vi "eventMode.vi"() -> ()   [LabVIEW 2019]
uses:
  TypeDefs/pixArrSmol.ctl
  <vilib>/Math Plots/3D Math Plots/3D Surface/3D Surface XCtrl/3D Surface.xctl
  <vilib>/Instr/_visa.llb/VISA Flush IO Buffer Mask.ctl
  <extravilib>/ChannelInstances/Tag-bool/Read With Abort.vi
  <extravilib>/ChannelInstances/Tag-bool/Write With Abort.vi
  <extravilib>/ChannelInstances/Tag-bool/Instantiate.vi
  <extravilib>/ChannelInstances/Tag-bool/EndpointRead.vi
  <extravilib>/ChannelInstances/Tag-bool/Endpoint.vi
  <vilib>/Instr/_visa.llb/VISA Configure Serial Port (Instr).vi
  <extravilib>/ChannelInstances/Tag-bool.lvlib
  TypeDefs/serialSettings_Global.vi
panel:
  in  "Reset EEPROM":bool
  in  "Update EEPROM":bool
  in  "Serial Settings":T1={"VISA resource name"="COM6", "baud rate"=115200, "data bits"=8, "parity"=enum."None", "stop bits"=10, "flow control"=0} {"baud rate" items=["75"=75, "110"=110, "134"=134, "150"=150, "300"=300, "600"=600, "1200"=1200, "1800"=1800, "2400"=2400, "4800"=4800, "7200"=7200, "9600"=9600, "14400"=14400, "19200"=19200, "28800"=28800, "38400"=38400, "56000"=56000, "57600"=57600, "115200"=115200, "128000"=128000, "230400"=230400]; "stop bits" items=["1.0"=10, "1.5"=15, "2.0"=20]; "flow control" items=["None"=0, "XON/XOFF"=1, "RTS/CTS"=2, "DTR/DSR"=4]}
  out "Serial2 Same?":bool caption="Match 2?"
  out "Serial1 Same?":bool caption="Match?"
  in  "CZT 2 Serial In":u32 caption="Enter CZT 2 Serial Number"
  out "CZT 2 Serial":sgl=nan
  in  "CZT 1 Serial In":u32 caption="Enter CZT 1 Serial Number"
  out "CZT 1 Serial":sgl=nan
  in  "Clear Serial":bool
  in  "Read Serial":bool
  in  "Iteration Limit":u32=4999
  out "Exit error code":errorcluster
  in  "Event Counts":enum32{"3D Surface ", "Histogram", "Heat Map"}(tab)
  out "Detector Surface":refnum<class "3D Plot Datatype.lvclass">[](xcontrol)
  out "Event Count Histogram":T2(graph)
  out "Intensity Graph":u32[][](graph)
  out "Energy Spectrum":T2(graph)
  out "Input Size":i32[](array[numeric])
  out "All rows":string[][](array[string])
  out "Clean No Dups Size":i32[](array[numeric])
  out "Clean+No Dups":string[][](array[string])
  in  "Select CZT":enum32{"CZT 1", "CZT 2"}(radio)
  in  "PixOff":bool
  in  "Get All Pixel Status":bool
  out "Column":u8=1
  out "Row":string="A"
  in  "PixOn":bool
  in  "Choose Pixel":u8 format="%02.0f"
  in  "CZT Tabs":enum32{"CZT 1", "CZT 2"}(tab)=enum."CZT 2"
  out "Pixel Status 1":T3=[[TRUE, TRUE, TRUE, TRUE, TRUE, TRUE, TRUE, TRUE, TRUE, TRUE, TRUE, TRUE, TRUE, TRUE, TRUE, TRUE, TRUE], [TRUE, TRUE, TRUE, TRUE, TRUE, TRUE, TRUE, TRUE, TRUE, TRUE, TRUE, TRUE, TRUE, TRUE, TRUE, TRUE, TRUE], [TRUE, TRUE, TRUE, TRUE, TRUE, TRUE, TRUE, TRUE, TRUE, TRUE, TRUE, TRUE, TRUE, TRUE, TRUE, TRUE, TRUE], [TRUE, TRUE, TRUE, TRUE, TRUE, TRUE, TRUE, TRUE, TRUE, TRUE, TRUE, TRUE, TRUE, TRUE, TRUE, TRUE, TRUE], [TRUE, TRUE, TRUE, TRUE, TRUE, TRUE, TRUE, TRUE, TRUE, TRUE, TRUE, TRUE, TRUE, TRUE, TRUE, TRUE, TRUE], [TRUE, TRUE, TRUE, TRUE, TRUE, TRUE, TRUE, TRUE, TRUE, TRUE, TRUE, TRUE, TRUE, TRUE, TRUE, TRUE, TRUE], [TRUE, TRUE, TRUE, TRUE, TRUE, TRUE, TRUE, TRUE, TRUE, TRUE, TRUE, TRUE, TRUE, TRUE, TRUE, TRUE, TRUE], [TRUE, TRUE, TRUE, TRUE, TRUE, TRUE, TRUE, TRUE, TRUE, TRUE, TRUE, TRUE, TRUE, TRUE, TRUE, TRUE, TRUE], [TRUE, TRUE, TRUE, TRUE, TRUE, TRUE, TRUE, TRUE, TRUE, TRUE, TRUE, TRUE, TRUE, TRUE, TRUE, TRUE, TRUE], [TRUE, TRUE, TRUE, TRUE, TRUE, TRUE, TRUE, TRUE, TRUE, TRUE, TRUE, TRUE, TRUE, TRUE, TRUE, TRUE, TRUE], [TRUE, TRUE, TRUE, TRUE, TRUE, TRUE, TRUE, TRUE, TRUE, TRUE, TRUE, TRUE, TRUE, TRUE, TRUE, TRUE, TRUE], [TRUE, TRUE, TRUE, TRUE, TRUE, TRUE, TRUE, TRUE, TRUE, TRUE, TRUE, TRUE, TRUE, TRUE, TRUE, TRUE, TRUE], [TRUE, TRUE, TRUE, TRUE, TRUE, TRUE, TRUE, TRUE, TRUE, TRUE, TRUE, TRUE, TRUE, TRUE, TRUE, TRUE, TRUE], [TRUE, TRUE, TRUE, TRUE, TRUE, TRUE, TRUE, TRUE, TRUE, TRUE, TRUE, TRUE, TRUE, TRUE, TRUE, TRUE, TRUE], [TRUE, TRUE, TRUE, TRUE, TRUE, TRUE, TRUE, TRUE, TRUE, TRUE, TRUE, TRUE, TRUE, TRUE, TRUE, TRUE, TRUE], [TRUE, TRUE, TRUE, TRUE, TRUE, TRUE, TRUE, TRUE, TRUE, TRUE, TRUE, TRUE, TRUE, TRUE, TRUE, TRUE, TRUE]]
  out "Pixel Status 2":T3=[[TRUE, TRUE, TRUE, TRUE, TRUE, TRUE, TRUE, TRUE, TRUE, TRUE, TRUE, TRUE, TRUE, TRUE, TRUE, TRUE, TRUE], [TRUE, TRUE, TRUE, TRUE, TRUE, TRUE, TRUE, TRUE, TRUE, TRUE, TRUE, TRUE, TRUE, TRUE, TRUE, TRUE, TRUE], [TRUE, TRUE, TRUE, TRUE, TRUE, TRUE, TRUE, TRUE, TRUE, TRUE, TRUE, TRUE, TRUE, TRUE, TRUE, TRUE, TRUE], [TRUE, TRUE, TRUE, TRUE, TRUE, TRUE, TRUE, TRUE, TRUE, TRUE, TRUE, TRUE, TRUE, TRUE, TRUE, TRUE, TRUE], [TRUE, TRUE, TRUE, TRUE, TRUE, TRUE, TRUE, TRUE, TRUE, TRUE, TRUE, TRUE, TRUE, TRUE, TRUE, TRUE, TRUE], [TRUE, TRUE, TRUE, TRUE, TRUE, TRUE, TRUE, TRUE, TRUE, TRUE, TRUE, TRUE, TRUE, TRUE, TRUE, TRUE, TRUE], [TRUE, TRUE, TRUE, TRUE, TRUE, TRUE, TRUE, TRUE, TRUE, TRUE, TRUE, TRUE, TRUE, TRUE, TRUE, TRUE, TRUE], [TRUE, TRUE, TRUE, TRUE, TRUE, TRUE, TRUE, TRUE, TRUE, TRUE, TRUE, TRUE, TRUE, TRUE, TRUE, TRUE, TRUE], [TRUE, TRUE, TRUE, TRUE, TRUE, TRUE, TRUE, TRUE, TRUE, TRUE, TRUE, TRUE, TRUE, TRUE, TRUE, TRUE, TRUE], [TRUE, TRUE, TRUE, TRUE, TRUE, TRUE, TRUE, TRUE, TRUE, TRUE, TRUE, TRUE, TRUE, TRUE, TRUE, TRUE, TRUE], [TRUE, TRUE, TRUE, TRUE, TRUE, TRUE, TRUE, TRUE, TRUE, TRUE, TRUE, TRUE, TRUE, TRUE, TRUE, TRUE, TRUE], [TRUE, TRUE, TRUE, TRUE, TRUE, TRUE, TRUE, TRUE, TRUE, TRUE, TRUE, TRUE, TRUE, TRUE, TRUE, TRUE, TRUE], [TRUE, TRUE, TRUE, TRUE, TRUE, TRUE, TRUE, TRUE, TRUE, TRUE, TRUE, TRUE, TRUE, TRUE, TRUE, TRUE, TRUE], [TRUE, TRUE, TRUE, TRUE, TRUE, TRUE, TRUE, TRUE, TRUE, TRUE, TRUE, TRUE, TRUE, TRUE, TRUE, TRUE, TRUE], [TRUE, TRUE, TRUE, TRUE, TRUE, TRUE, TRUE, TRUE, TRUE, TRUE, TRUE, TRUE, TRUE, TRUE, TRUE, TRUE, TRUE], [TRUE, TRUE, TRUE, TRUE, TRUE, TRUE, TRUE, TRUE, TRUE, TRUE, TRUE, TRUE, TRUE, TRUE, TRUE, TRUE, TRUE]]
  out "Noisy Pixel List":i32[][](array[numeric])
  in  "Open CSV":bool
  out "States Left":string
  out "Current Time":timestamp format="%<%x\n%X>T"
  out "CZT 2 \nFrequency":u8 format="%d Mhz"
  in  "Set Clock":bool
  in  "Set CZT Clock":u8(ring)=2 items=["30 Mhz"=6, "25 Mhz"=5, "20 Mhz"=4, "15 Mhz"=3, "10 Mhz"=2]
  out "CZT 1\nFrequency":u8 format="%d Mhz"
  out "CZT 2 Thresh":u16 format="%u KeV"
  in  "Select Threshold Value":u16(slide)=20 min=20 max=200 scale=20.0..200.0
  in  "Set Threshold":bool
  out "CZT 1 Thresh":u16 format="%u KeV"
  in  "Test Description":string caption="(Inserted in FITS header)"
  in  "Stop":bool
  in  "Start Event":bool
  in  "Short Description":string caption="(Appended to file name)"
  in  "User Name":string
  in  "Acquisition Period":T4={"Hours"=0, "Minutes"=0, "Seconds"=10}
  out "Event Mode":bool
  out "Events Count":u32
  out "FITS File":bool
  out "Time elapsed":dbl format="%<%H:%M:%S>t"
  in  "Exit":bool
  # "Event Mode Test"
  # "Event Start:    A0FF55\nEvent Stop:    A00055\nEmu +Eve :    A1FF55\nRead Serial:   BXXX55\nClock Set  :    C00X55\nThresh Set:    EXXX55\nUpdate EE:     F00155\nReset EE   :     F00055"
  # "Pix On  CZT1: D0XX55\nPix Off  CZT1: D1XX55\nPix On  CZT2: D2XX55\nPix Off  CZT2: D3XX55\nChck All Pix  : DFXX55"
  # "Pixel Matrix Settings"
  # "Channel"
  # "Counts"
  # "Energy Threshold Settings"
  # "KeV"
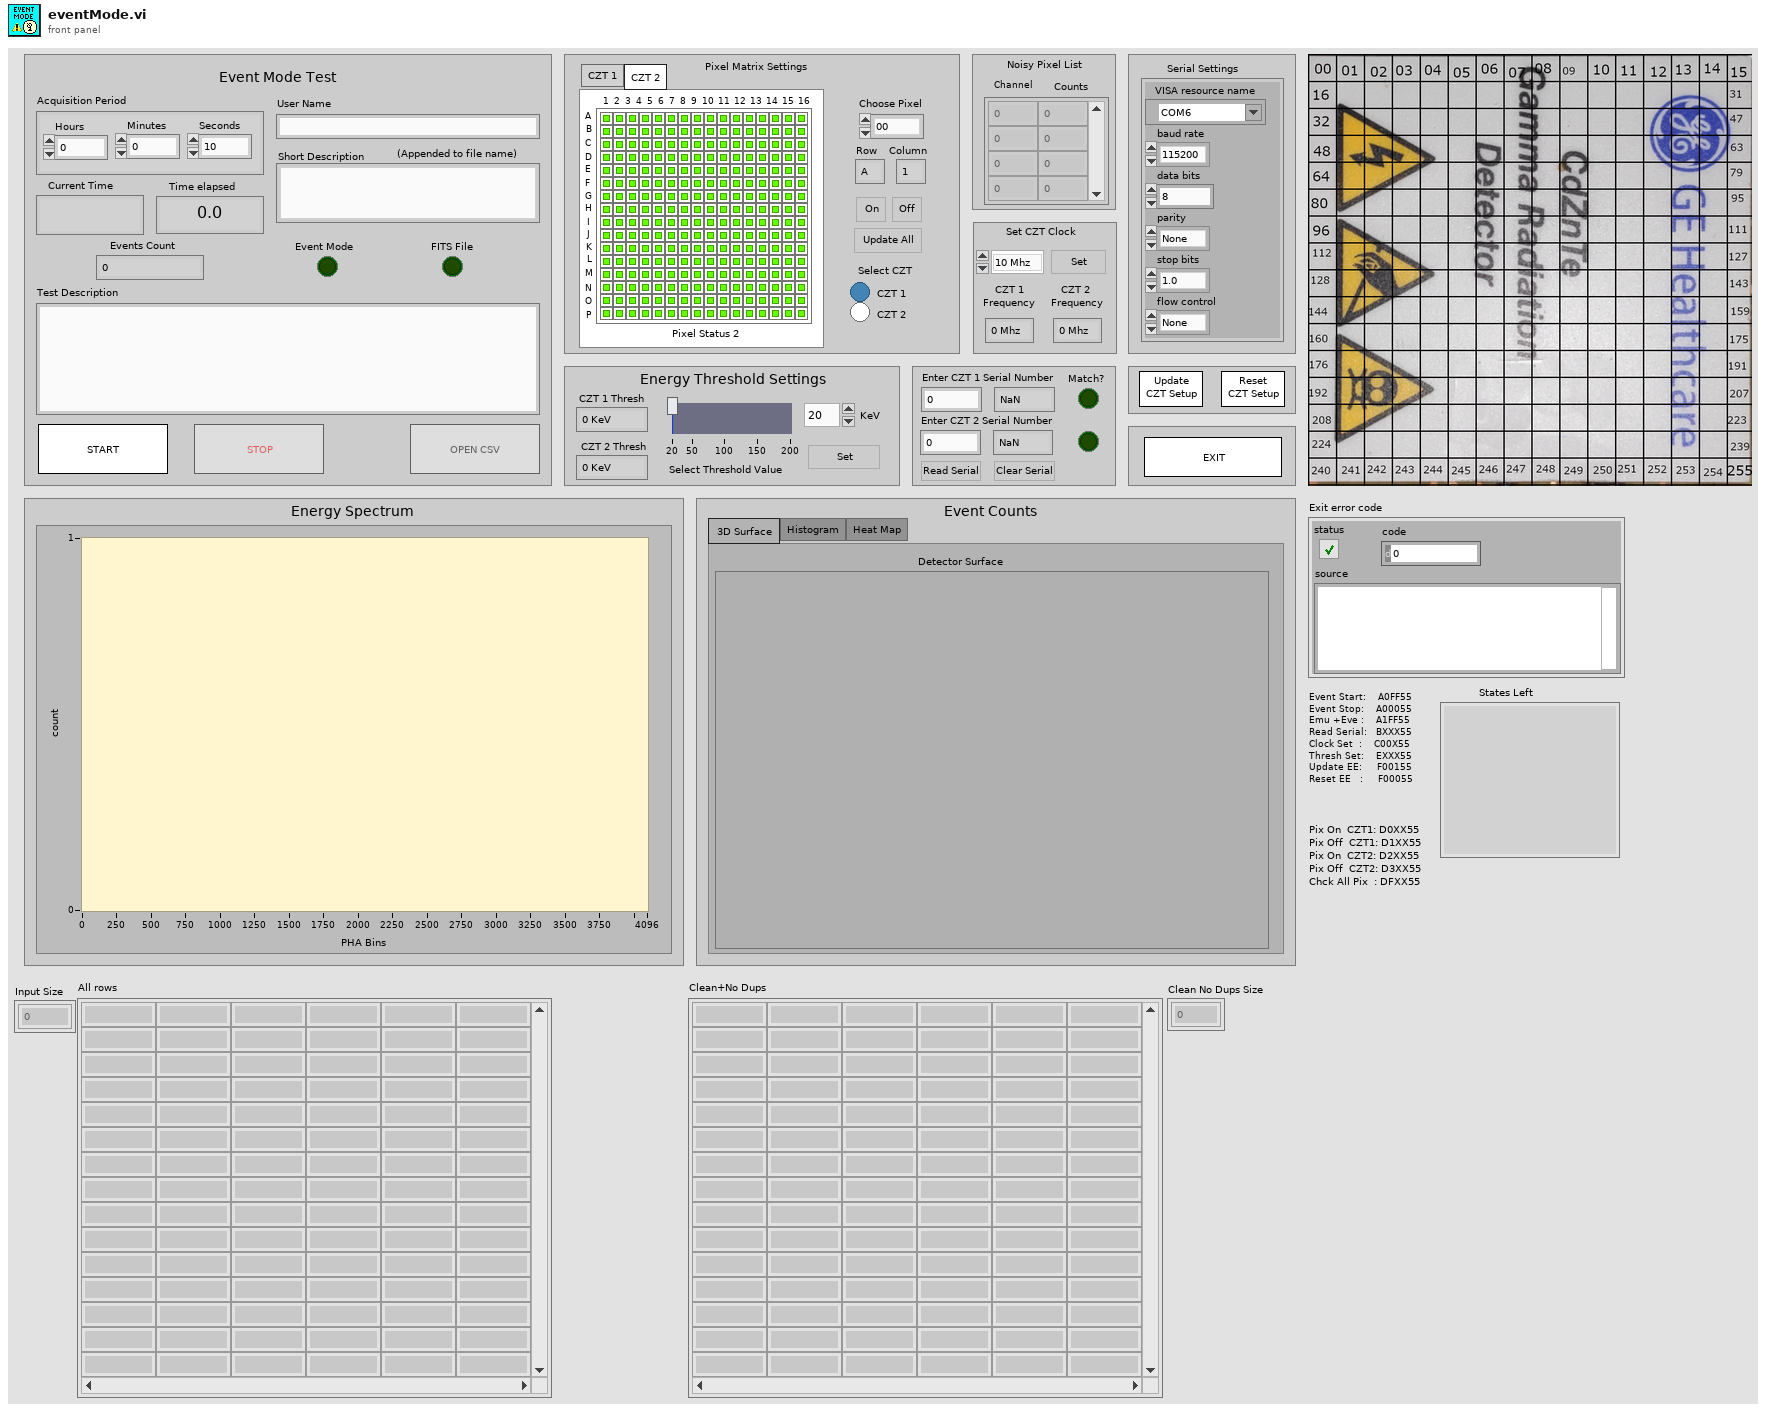
[diagram p1: front panel]
types:
  T1 = cluster{"VISA resource name":refnum<visa-resource-name>, "baud rate":u32, "data bits":u16, "parity":enum16{"None", "Odd", "Even", "Mark", "Space"}, "stop bits":u16, "flow control":u16}
  T2 = cluster{"X Values":dbl[], "Histogram: h(x)":i32[]}
  T3 = typedef "pixArrSmol.ctl" = bool[][]
  T4 = cluster{"Hours":u32, "Minutes":u32, "Seconds":u32}
  T5 = enum32{"Invalid", "Standard", "Closed", "Hidden", "Minimized", "Maximized"}
  T6 = enum32{"invalid app kind", "Development System", "Run Time System", "Student Edition", "Embedded LabVIEW", "Evaluation", "Custom"}
  T7 = enum8{"Enabled", "Disabled", "Disabled and Grayed Out"}
  T8 = typedef "Tag-bool.lvlib/))Channel.ctl" = refnum<queue>
  T9 = cluster{"Core":cluster{"Current VI Reference":refnum<vi>, "Close Panel on Exit?":bool}, "Stop Pressed?":bool, "Start Time":dbl, "Acquisition Period":dbl, "Iteration Count":u32, "CSV File Data":cluster{"Dump txt file path":path, "Data Buffer":string, "Valid Data in Buffer":i32, "CSV file path":path, "Fits File name":string, "Test Start time":timestamp}, "User & Config Data":cluster{"User Name":string, "Short Description":string, "Description":string, "CZT Threshold 1":u16, "CZT Threshold 2":u16}, "Pixel Status 1":cluster{"Pixel Number":u16, "Pixel En/Dis?":bool, "Pixel Array":bool[][], "Disabled Pixels":u8[]}, "Pixel Status 2":cluster{"Pixel Number":u16, "Pixel En/Dis?":bool, "Pixel Array":bool[][], "Disabled Pixels":u8[]}}
  T10 = cluster{"Pixel Number":u16, "Pixel En/Dis?":bool, "Pixel Array":bool[][], "Disabled Pixels":u8[]}
  T11 = cluster{"User Name":string, "Short Description":string, "Description":string, "CZT Threshold 1":u16, "CZT Threshold 2":u16}
  T12 = cluster{"Dump txt file path":path, "Data Buffer":string, "Valid Data in Buffer":i32, "CSV file path":path, "Fits File name":string, "Test Start time":timestamp}
  T13 = cluster{"Current VI Reference":refnum<vi>, "Close Panel on Exit?":bool}
  T14 = cluster{"User Name":string, "Short Description ":string, "Test Description":string, "Value":u16, "Value":u16}
  T15 = cluster{"Dump txt file path":path, "Data buffer OUT":string, "Valid Data Buf OUT":i32, "CSV file path":path, "Fits File name":string, "Test Start time":timestamp}
  T16 = typedef "VISA Flush IO Buffer Mask.ctl" = u16
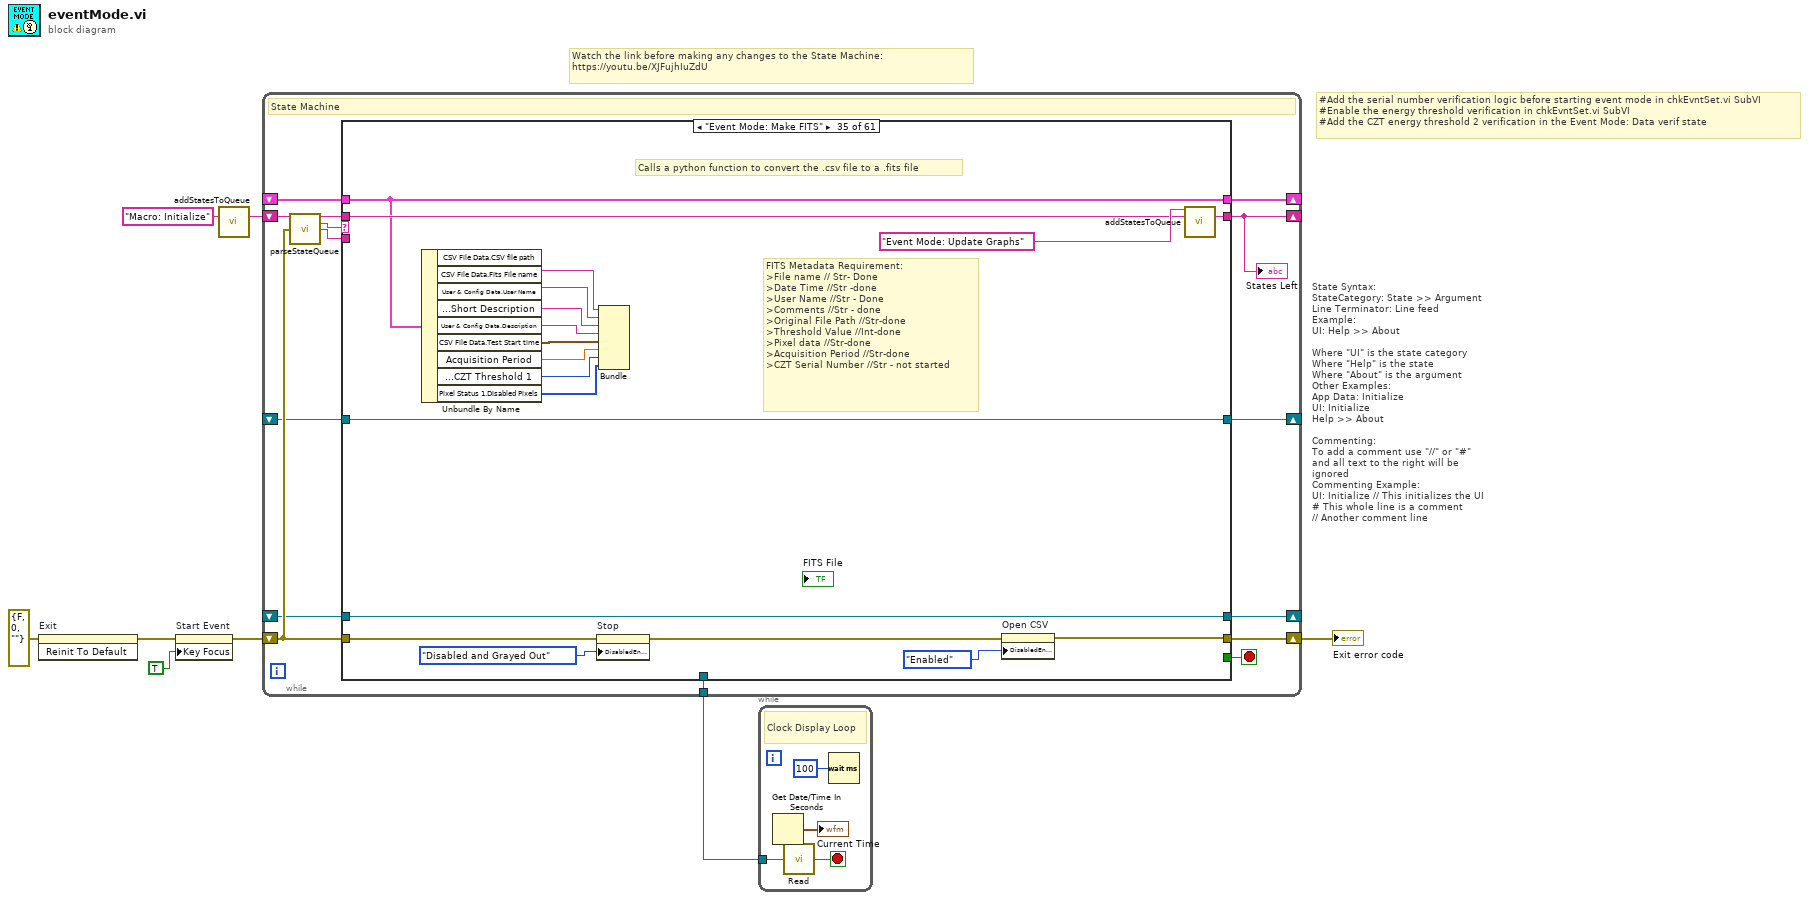
[diagram p0: block diagram]
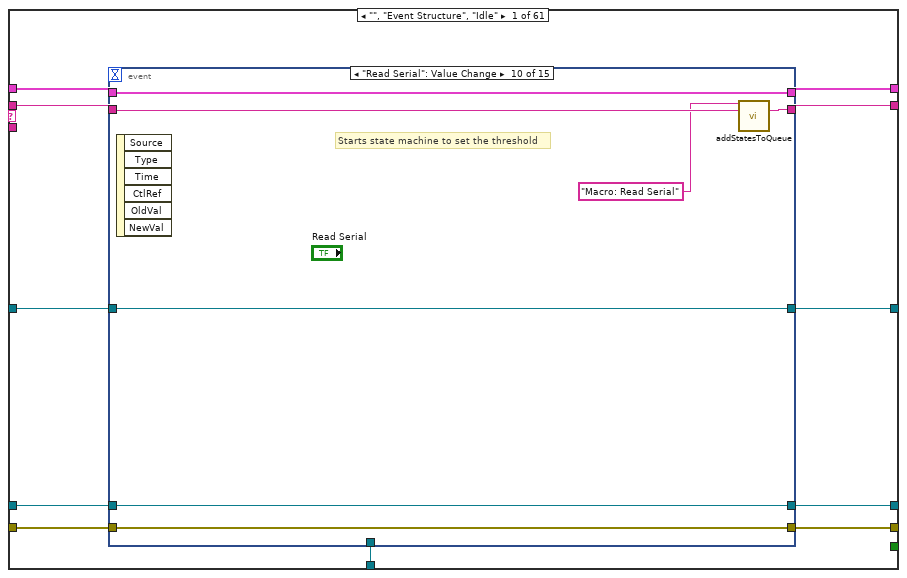
[diagram p2: hidden frame]
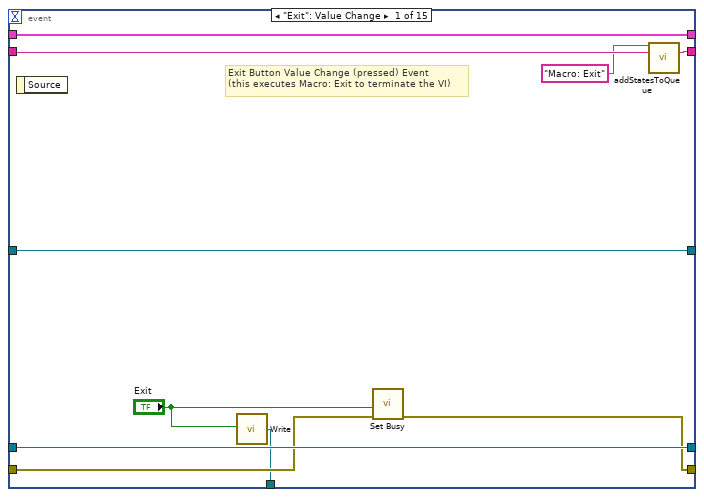
[diagram p3: hidden frame]
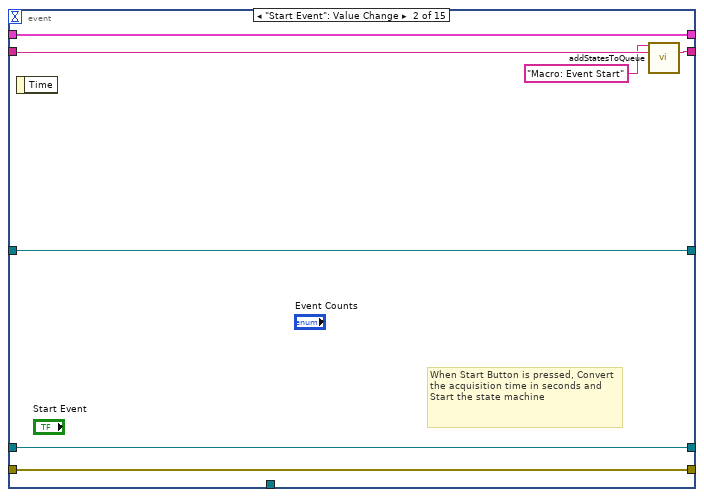
[diagram p4: hidden frame]
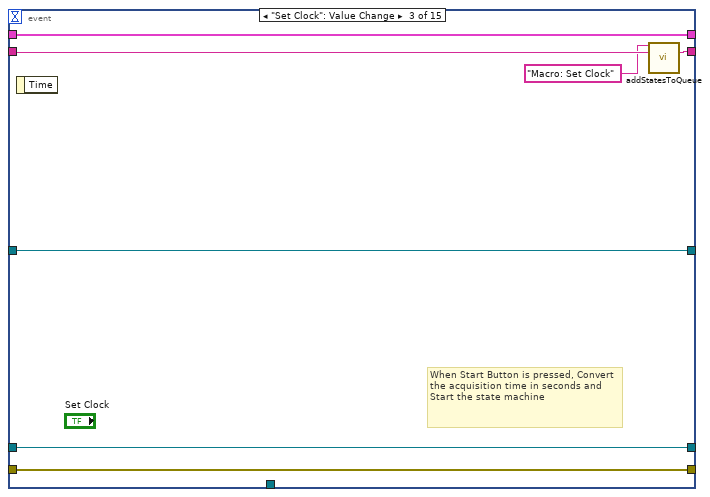
[diagram p5: hidden frame]
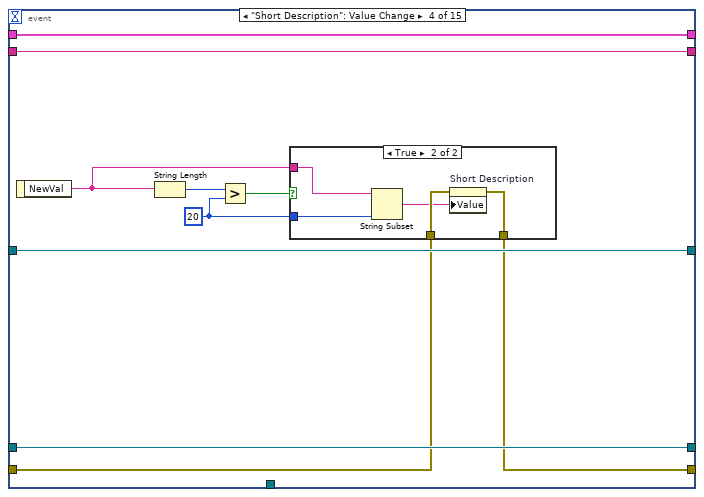
[diagram p6: hidden frame]
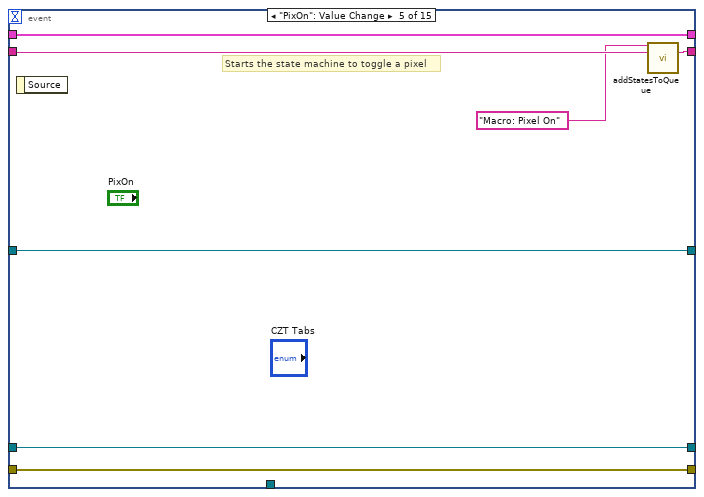
[diagram p8: hidden frame]
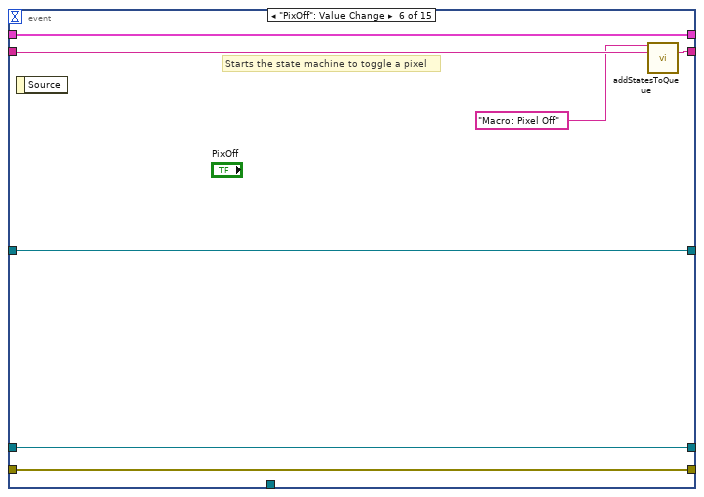
[diagram p9: hidden frame]
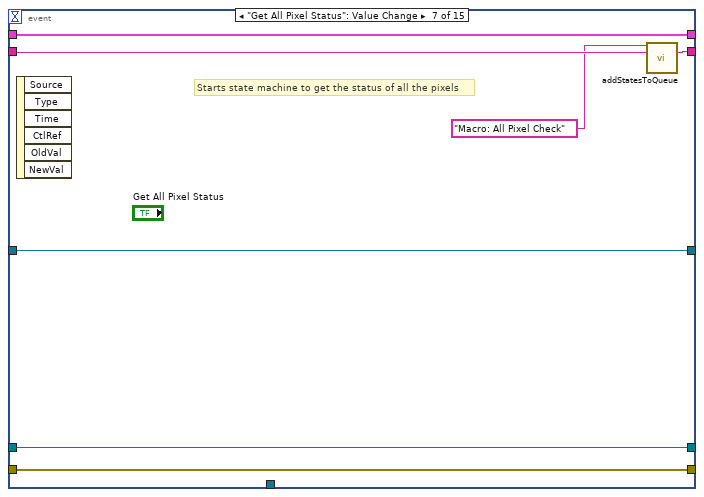
[diagram p10: hidden frame]
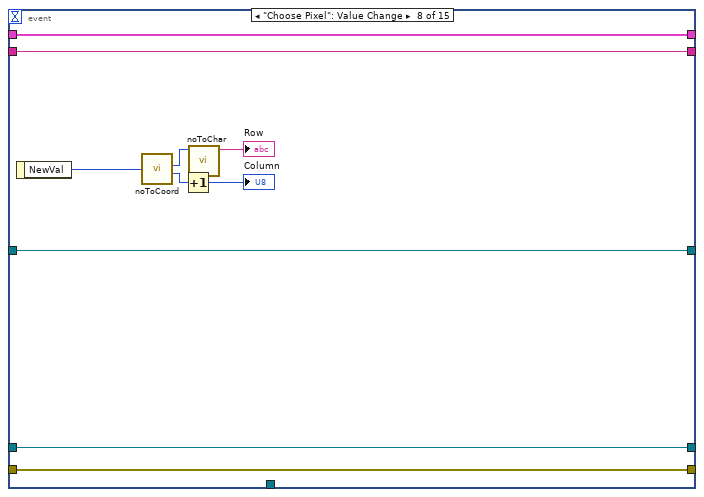
[diagram p11: hidden frame]
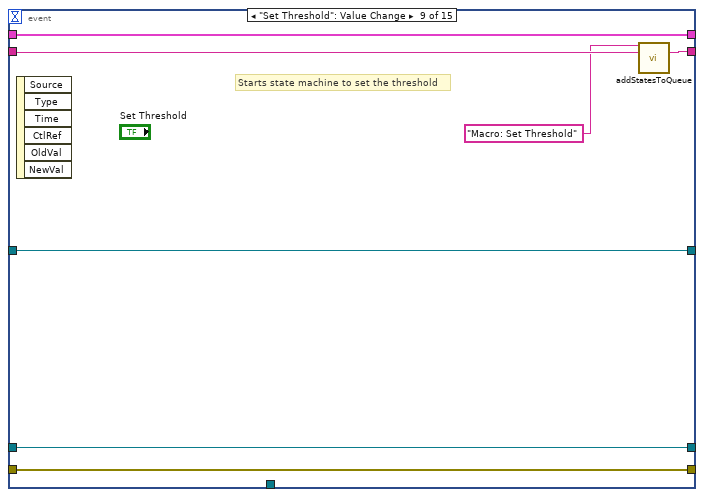
[diagram p12: hidden frame]
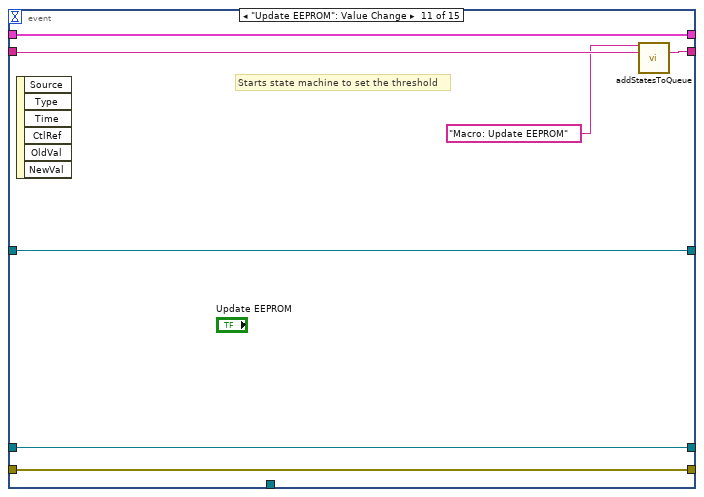
[diagram p13: hidden frame]
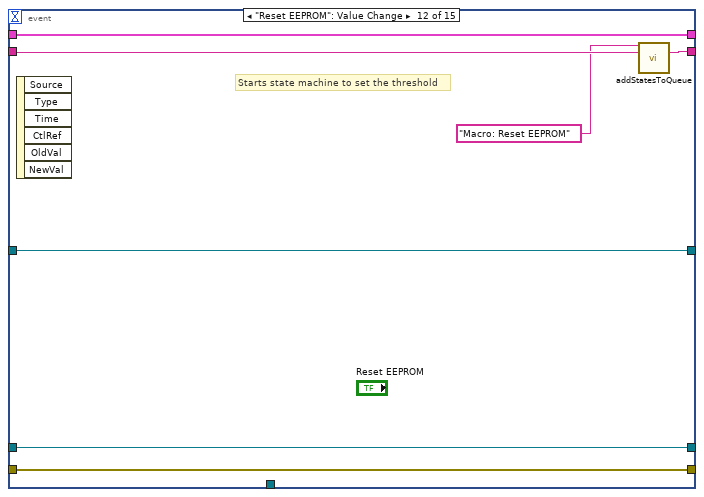
[diagram p14: hidden frame]
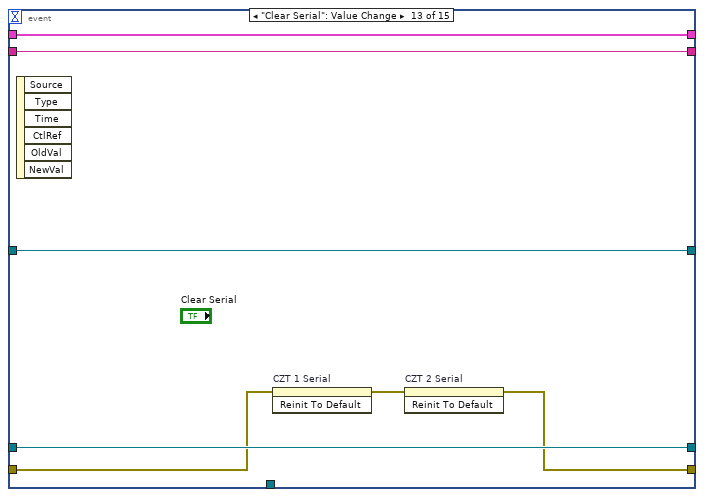
[diagram p15: hidden frame]
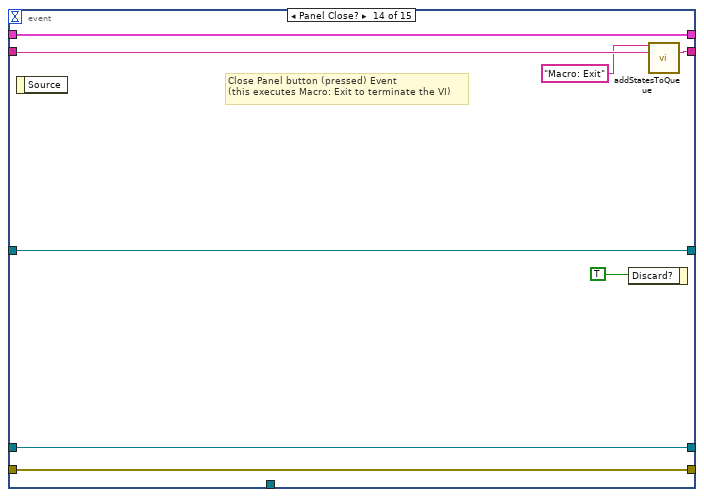
[diagram p16: hidden frame]
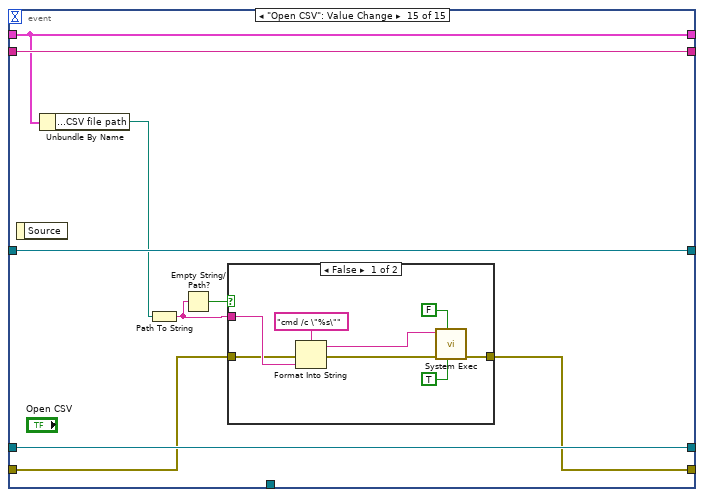
[diagram p17: hidden frame]
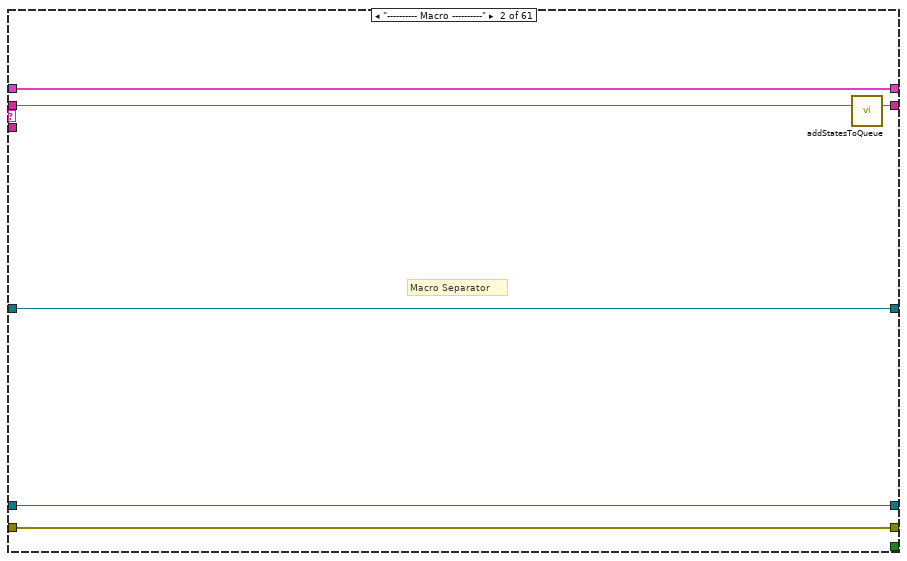
[diagram p19: hidden frame]
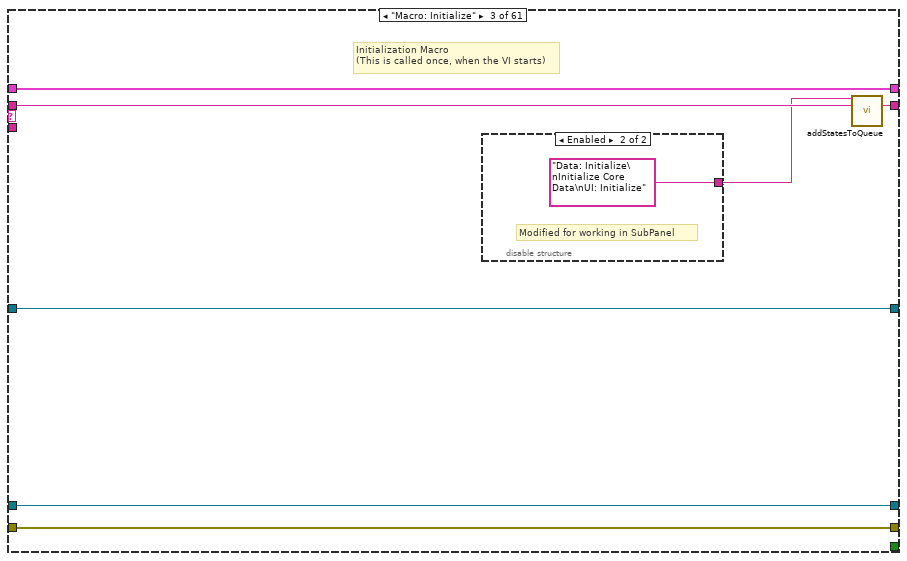
[diagram p20: hidden frame]
diagram:
  # "#Add the serial number verification logic before starting event mode in chkEvntSet.vi SubVI\n#Enable the energy threshold verification in chkEvntSet.vi SubVI\n#Add the CZT energy threshold 2 verification in the Event Mode: Data verif state"
  # "Watch the link before making any changes to the State Machine:\nhttps://youtu.be/XJFujhIuZdU"
  # "State Syntax:\nStateCategory: State >> Argument\nLine Terminator: Line feed\nExample:\nUI: Help >> About\n\nWhere \"UI\" is the state category\nWhere \"Help\" is the state\nWhere \"About\" is the argument\nOther Examples:\nApp Data: Initialize\nUI: Initialize\nHelp >> About\n\nCommenting:\nTo add a comment use \"//\" or \"#\" and all text to the right will be ignored\nCommenting Example:\nUI: Initialize // This initializes the UI\n# This whole line is a comment\n// Another comment line"
  n1 = invoke on="Exit" class="Bool (strict)" method="Reinit To Default"(error in=errorcluster {"status"=FALSE, "code"=0, "source"=""} ("error in (no error)")) -> (error out=w3:errorcluster)  [unwired: 2 in, 2 out]
  n2 = property on="Start Event" class="Bool"(error in=w3, "Key Focus"=TRUE) -> (error out=w2:errorcluster)  [unwired: 1 in, 1 out]
  n3 = call "addStatesToQueue.vi"("State(s) in (\"\")"="Macro: Initialize") -> ("States Out"=w8:string)  [unwired: 14 in]
  n4 = while "JKI State Machine 2018" {
    shift-right: [w17] -> _
    shift-left: _ -> [w16]
    shift-right: [w19] -> w5
    shift-left: w2 -> [w15]
    shift-right: [w18] -> _
    shift-left: w8 -> [w20]
    shift-right: [w14] -> _
    shift-left: _ -> [w13]
    shift-right: [w12] -> _
    shift-left: _ -> [w11]
    tunnel: [w9] -> w4
    stop <- w10 stop-if-true
    # "State Machine"
    n5 = call "parseStateQueue.vi"("State Queue"=w20, "Error In (no error)"=w15) -> ("Remaining States"=w22:string, "Current State"=w23:string, "Arguments"=w21:string)  [unwired: 11 in]
    n6 = case shown="\"Event Mode: Make FITS\"" w23 {
      selector: w23 -> [_ _ _ _ _ _ _ _ _ _ _ _ _ _ w265 _ _ _ _ _ _ _ _ _ _ _ _ _ _ _ _ _ _ _ _ _ _ _ _ _ _ _ _ _ _ _ _ _ _ _ _ _ _ _ _ _ _ _ _ _ _]
      tunnel: w22 -> [w34 w172 w179 w188 w195 w202 w209 w216 w223 w230 w237 w244 w256 w262 w269 w290 w302 w319 w325 w331 w337 w352 w360 w366 w405 w413 w426 w497 w514 w536 w544 w564 w611 w691 w697 w734 w740 w760 w782 w805 w823 w853 w862 w885 w915 w921 w934 w955 w961 w974 w996 w1013 w1019 w1035 w1061 w1067 w1076 w1085 w1091 w1111 w1129]
      tunnel: w21 -> [_ _ _ _ _ _ _ _ _ _ _ _ _ _ _ _ _ _ _ _ _ _ _ _ _ w408 w420 _ _ _ _ _ _ w666 _ _ _ _ _ _ _ _ _ _ _ _ _ w945 _ _ w986 w1007 _ _ w1051 _ _ _ _ w1097 w1116]
      tunnel: w16 -> [w32 w169 w176 w185 w192 w199 w206 w213 w220 w227 w234 w241 w253 w259 w267 w283 w309 w317 w322 w328 w334 _ w355 w363 w403 w411 w422 w494 w505 w524 w550 w557 w601 w682 w696 w729 w737 w758 w780 w798 w820 w850 w860 w879 w905 w918 w932 w953 w958 w972 w994 w1011 w1016 w1033 w1059 w1064 w1074 w1083 w1088 w1109 w1127]
      tunnel: [w31 w170 w177 w186 w193 w200 w207 w214 w221 w228 w235 w242 w254 w260 w271 w287 errorcluster {"status"=FALSE, "code"=0, "source"=""} ("error out") w313 w323 w329 w335 w349 w356 w364 w384 w409 w423 w495 w500 w521 w539 w556 w605 w671 w698 w722 w738 w748 w768 w788 w817 w851 w855 w871 w887 w919 w927 w941 w959 w969 w989 w997 w1017 w1030 w1054 w1065 w1071 w1080 w1089 w1095 w1117] -> w19
      tunnel: w15 -> [w30 w170 w177 w186 w193 w200 w207 w214 w221 w228 w235 w242 w254 w260 w270 w287 w294 w314 w323 w329 w335 w349 w357 w364 w373 w410 w424 w495 w503 w518 w551 w555 w607 w674 w701 w727 w738 w747 w772 w800 w818 w851 w856 w880 w903 w919 w923 w949 w959 w964 w990 w1005 w1017 w1026 w1055 w1065 w1068 w1078 w1089 w1108 w1123]
      tunnel: [w33 w171 w178 w187 w194 w201 w208 w215 w222 w229 w236 w243 w255 w261 w268 w289 w311 w318 w324 w330 w336 w351 w359 w365 w404 w412 w425 w496 w513 w535 w552 w563 w610 w690 w714 w733 w739 w759 w781 w804 w822 w852 w861 w884 w914 w920 w933 w954 w960 w973 w995 w1012 w1018 w1034 w1060 w1066 w1075 w1084 w1090 w1110 w1128] -> w18
      tunnel: [_ _ _ _ _ _ _ _ _ _ _ _ _ _ _ _ _ TRUE _ _ _ _ _ _ _ _ _ _ _ _ _ _ _ _ _ _ _ _ _ _ _ _ _ _ _ _ _ _ _ _ _ _ _ _ _ _ _ _ _ _ _] -> w10
      tunnel: [w29 w169 w176 w185 w192 w199 w206 w213 w220 w227 w234 w241 w253 w259 w267 w288 w309 w317 w322 w328 w334 w350 w355 w363 w403 w411 w422 w494 w504 w523 w550 w560 w602 w681 w696 w729 w737 w758 w780 w799 w819 w850 w860 w878 w904 w918 w932 w953 w958 w972 w994 w1011 w1016 w1033 w1059 w1064 w1074 w1083 w1088 w1109 w1127] -> w17
      tunnel: [w25 w167 w173 w182 w190 w197 w204 w210 w217 w225 w232 w239 w245 w257 w263 w276 w308 w315 w320 w326 w332 w340 w353 w361 w399 w406 w418 w492 w499 w522 w543 w561 w606 w673 w711 w731 w735 w751 w774 w801 w815 w848 w857 w882 w912 w916 w929 w950 w956 w970 w991 w1006 w1014 w1031 w1056 w1062 w1072 w1081 w1086 w1096 _] -> w14
      tunnel: w13 -> [w26 w167 w173 w182 w190 w197 w204 w210 w217 w225 w232 w239 w245 w257 w263 w276 w308 w315 w320 w326 w332 w340 w353 w361 w399 w406 w418 w492 w499 w522 w543 w562 w608 w675 w711 w731 w735 w756 w778 w802 w816 w848 w858 w881 w912 w916 w922 w951 w956 w966 w992 w1006 w1014 w1027 w1057 w1062 w1070 w1079 w1086 _ w1125]
      tunnel: [w27 w168 w174 w184 w191 w198 w205 w212 w219 w226 w233 w240 w246 w258 w264 w277 w291 w316 w321 w327 w333 w345 w354 w362 w402 w407 w419 w493 w512 w534 w549 w558 w603 _ w713 w732 w736 w757 w779 w803 w821 w849 w859 w883 w913 w917 w931 w952 w957 w971 w993 w1010 w1015 w1032 w1058 w1063 w1073 w1082 w1087 w1098 w1126] -> w12
      tunnel: w11 -> [w28 w168 w174 w184 w191 w198 w205 w212 w219 w226 w233 w240 w246 w258 w264 w277 w291 w316 w321 w327 w333 w345 w354 w362 w402 w407 w419 w493 w512 w534 w549 _ w604 w688 w713 w732 w736 w757 w779 w803 w821 w849 w859 w883 w913 w917 w931 w952 w957 w971 w993 w1010 w1015 w1032 w1058 w1063 w1073 w1082 w1087 w1098 w1126]
      tunnel: [w24 _ _ _ _ _ _ _ _ _ _ _ _ _ _ _ _ _ _ _ _ _ _ _ _ _ _ _ _ _ _ _ _ _ _ _ _ _ _ _ _ _ _ _ _ _ _ _ _ _ _ _ _ _ _ _ _ _ _ _ _] -> w9
      frame "", "Event Structure", "Idle" {
        n7 = event shown="[9] \"Read Serial\": Value Change" {
          selector: _ -> [_ _ _ _ _ _ _ _ _ _ _ _ _ _ _]
          dyn-events: _ -> [_ _ _ _ _ _ _ _ _ _ _ _ _ _ _]
          timeout: _ -> [_ _ _ _ _ _ _ _ _ _ _ _ _ _ _]
          tunnel: w34 -> [w44 w51 w58 w65 w78 w85 w93 w103 w110 w117 w124 w131 w137 w148 w155]
          tunnel: [w43 w50 w57 w65 w79 w86 w92 w103 w109 w116 w123 w130 w137 w147 w155] -> w33
          tunnel: w32 -> [w42 w47 w54 w66 w80 w87 w94 w104 w111 w118 w125 w132 w138 w145 w154]
          tunnel: [w37 w46 w53 w63 w77 w84 w91 w102 w108 w115 w122 w129 w134 w146 w152] -> w31
          tunnel: w30 -> [w38 w46 w53 w64 w77 w84 w91 w102 w108 w115 w122 w129 w136 w146 w151]
          tunnel: [w42 w47 w54 w66 w80 w87 w94 w104 w111 w118 w125 w132 w138 w145 w154] -> w29
          tunnel: [w40 w48 w55 w68 w81 w88 w95 w105 w112 w119 w126 w133 w140 w142 w157] -> w27
          tunnel: w28 -> [w40 w48 w55 w68 w81 w88 w95 w105 w112 w119 w126 w133 w140 w142 w157]
          tunnel: w26 -> [w39 w45 w52 w67 w75 w82 w89 w96 w106 w113 w120 w127 w139 w141 w156]
          tunnel: [w39 w45 w52 w67 w75 w82 w89 w96 w106 w113 w120 w127 w139 w141 w156] -> w25
          tunnel: [w35 _ _ _ _ _ _ _ _ _ _ _ _ _ _] -> w24
          event "Exit": Value Change {
            # "Exit Button Value Change (pressed) Event\n(this executes Macro: Exit to terminate the VI)"
            n8 = event-data() -> ()  [unwired: 1 in, 1 out]
            n9 = call <extravilib>:"Write.vi"("element"="Exit") -> ("channel"=w35:T8)  [unwired: 1 out]
            n10 = call <vilib>:"Set Busy.vi"("error in (no error)"=w38, "disable click? (T)"="Exit") -> ("error out"=w37:errorcluster)  [unwired: 8 in, 1 out]
            n11 = call "addStatesToQueue.vi"("State(s) in Front (\"\")"="Macro: Exit", "State(s) in (\"\")"=w44) -> ("States Out"=w43:string)  [unwired: 13 in]
          }
          event "Start Event": Value Change {
            # "When Start Button is pressed, Convert the acquisition time in seconds and Start the state machine"
            n12 = event-data() -> ()  [unwired: 1 in, 1 out]
            n13 = call "addStatesToQueue.vi"("State(s) in Front (\"\")"="Macro: Event Start", "State(s) in (\"\")"=w51) -> ("States Out"=w50:string)  [unwired: 13 in]
          }
          event "Set Clock": Value Change {
            # "When Start Button is pressed, Convert the acquisition time in seconds and Start the state machine"
            n14 = event-data() -> ()  [unwired: 1 in, 1 out]
            n15 = call "addStatesToQueue.vi"("State(s) in Front (\"\")"="Macro: Set Clock", "State(s) in (\"\")"=w58) -> ("States Out"=w57:string)  [unwired: 13 in]
          }
          event "Short Description": Value Change {
            w59 = 20
            n16 = event-data() -> ("NewVal"=w62:string)  [unwired: 1 in]
            n17 = String Length(string=w62) -> (length=w61:i32)
            n18 = Greater?(x=w61, y=w59) -> (0:w60:bool)
            n19 = case shown="True" w60 {
              tunnel: w64 -> [w69 w74]
              tunnel: [w69 w73] -> w63
              tunnel: w62 -> [_ w72]
              tunnel: w59 -> [_ w70]
              frame False {
              }
              frame True {
                n20 = String Subset(string=w72, length (rest)=w70) -> (substring=w71:string)  [unwired: 1 in]
                n21 = property on="Short Description" class="Str"(error in=w74, "Value"=w71) -> (error out=w73:errorcluster)  [unwired: 1 in, 1 out]
              }
            }
          }
          event "PixOn": Value Change {
            # "Starts the state machine to toggle a pixel"
            n22 = event-data() -> ()  [unwired: 1 in, 1 out]
            n23 = call "addStatesToQueue.vi"("State(s) in Front (\"\")"="Macro: Pixel On" ("State(s) in Front (\"\")"), "State(s) in (\"\")"=w78) -> ("States Out"=w79:string)  [unwired: 13 in]
          }
          event "PixOff": Value Change {
            # "Starts the state machine to toggle a pixel"
            n24 = event-data() -> ()  [unwired: 1 in, 1 out]
            n25 = call "addStatesToQueue.vi"("State(s) in Front (\"\")"="Macro: Pixel Off" ("State(s) in Front (\"\")"), "State(s) in (\"\")"=w85) -> ("States Out"=w86:string)  [unwired: 13 in]
          }
          event "Get All Pixel Status": Value Change {
            # "Starts state machine to get the status of all the pixels"
            n26 = event-data() -> ()  [unwired: 1 in, 6 out]
            n27 = call "addStatesToQueue.vi"("State(s) in Front (\"\")"="Macro: All Pixel Check" ("State(s) in Front (\"\")"), "State(s) in (\"\")"=w93) -> ("States Out"=w92:string)  [unwired: 13 in]
          }
          event "Choose Pixel": Value Change {
            n28 = event-data() -> ("NewVal"=w101:u8)  [unwired: 1 in]
            n29 = call "noToCoord.vi"("Pixel number"=w101) -> ("i"=w98:u8, "j"=w100:u8)  [unwired: 6 in]
            n30 = Increment(x=w100) -> (x+1=→"Column":u8)
            n31 = call "noToChar.vi"("i"=w98) -> ("String"=→"Row":string)  [unwired: 10 in]
          }
          event "Set Threshold": Value Change {
            # "Starts state machine to set the threshold"
            n32 = event-data() -> ()  [unwired: 1 in, 6 out]
            n33 = call "addStatesToQueue.vi"("State(s) in Front (\"\")"="Macro: Set Threshold" ("State(s) in Front (\"\")"), "State(s) in (\"\")"=w110) -> ("States Out"=w109:string)  [unwired: 13 in]
          }
          event "Read Serial": Value Change {
            # "Starts state machine to set the threshold"
            n34 = event-data() -> ()  [unwired: 1 in, 6 out]
            n35 = call "addStatesToQueue.vi"("State(s) in Front (\"\")"="Macro: Read Serial" ("State(s) in Front (\"\")"), "State(s) in (\"\")"=w117) -> ("States Out"=w116:string)  [unwired: 13 in]
          }
          event "Update EEPROM": Value Change {
            # "Starts state machine to set the threshold"
            n36 = event-data() -> ()  [unwired: 1 in, 6 out]
            n37 = call "addStatesToQueue.vi"("State(s) in Front (\"\")"="Macro: Update EEPROM" ("State(s) in Front (\"\")"), "State(s) in (\"\")"=w124) -> ("States Out"=w123:string)  [unwired: 13 in]
          }
          event "Reset EEPROM": Value Change {
            # "Starts state machine to set the threshold"
            n38 = event-data() -> ()  [unwired: 1 in, 6 out]
            n39 = call "addStatesToQueue.vi"("State(s) in Front (\"\")"="Macro: Reset EEPROM" ("State(s) in Front (\"\")"), "State(s) in (\"\")"=w131) -> ("States Out"=w130:string)  [unwired: 13 in]
          }
          event "Clear Serial": Value Change {
            n40 = event-data() -> ()  [unwired: 1 in, 6 out]
            n41 = invoke on="CZT 1 Serial" class="DigNum (strict)" method="Reinit To Default"(error in=w136) -> (error out=w135:errorcluster)  [unwired: 2 in, 2 out]
            n42 = invoke on="CZT 2 Serial" class="DigNum (strict)" method="Reinit To Default"(error in=w135) -> (error out=w134:errorcluster)  [unwired: 2 in, 2 out]
          }
          event Panel Close? {
            # "Close Panel button (pressed) Event\n(this executes Macro: Exit to terminate the VI)"
            n43 = event-data() -> ()  [unwired: 1 in, 1 out]
            n44 = event-data("Discard?"=TRUE) -> ()  [unwired: 1 in, 1 out]
            n45 = call "addStatesToQueue.vi"("State(s) in Front (\"\")"="Macro: Exit", "State(s) in (\"\")"=w148) -> ("States Out"=w147:string)  [unwired: 13 in]
          }
          event "Open CSV": Value Change {
            n46 = event-data() -> ()  [unwired: 1 in, 1 out]
            n47 = Unbundle By Name(w154) -> ("CSV File Data.CSV file path"=w153:path)
            n48 = Path To String(path=w153) -> (string=w150:string)
            n49 = Empty String/Path?(string/path=w150) -> (empty?=w149:bool)
            n50 = case shown="False" w149 {
              tunnel: w150 -> [w165 _]
              tunnel: [w159 w166] -> w152
              tunnel: w151 -> [w158 w166]
              frame False {
                n51 = Format Into String(format string="cmd /c \"%s\"", error in=w158, w165) -> (resulting string=w163:string, error out=w164:errorcluster)  [unwired: 1 in]
                n52 = call <vilib>:"System Exec.vi"("run minimized? (F)"=TRUE ("run minimized?"), "wait until completion? (T)"=FALSE ("wait until completion?"), "error in (no error)"=w164, "command line"=w163) -> ("error out"=w159:errorcluster)  [unwired: 4 in, 3 out]
              }
              frame True {
              }
            }
          }
        }
      }
      frame "---------- Macro ----------" {
        # "Macro Separator"
        n53 = call "addStatesToQueue.vi"("State(s) in (\"\")"=w172) -> ("States Out"=w171:string)  [unwired: 14 in]
      }
      frame "Macro: Initialize" {
        # "Initialization Macro\n(This is called once, when the VI starts)"
        n54 = disable-structure shown="Enabled" {
          disable-tunnel: [w180 "Data: Initialize\nInitialize Core Data\nUI: Initialize"] -> w175
          frame Disabled {
            w180 = "Data: Initialize\nInitialize Core Data\nUI: Initialize\nUI: Front Panel State >> Standard"  # Data: Initialize Initialize Core Data UI: Initialize UI: Front Panel State >> Standard
          }
          frame Enabled {
            # "Modified for working in SubPanel"
          }
        }
        n55 = call "addStatesToQueue.vi"("State(s) in Front (\"\")"=w175, "State(s) in (\"\")"=w179) -> ("States Out"=w178:string)  [unwired: 13 in]
      }
      frame "Macro: Event Start" {
        n56 = call "addStatesToQueue.vi"("State(s) in Front (\"\")"="Event Mode: Data Init\nEvent Mode: Data Get\nEvent Mode: Data Verif\nUART Comm: Init >>Event Mode: Send Cmd", "State(s) in (\"\")"=w188) -> ("States Out"=w187:string)  [unwired: 13 in]
      }
      frame "Macro: Pixel On" {
        n57 = call "addStatesToQueue.vi"("State(s) in Front (\"\")"="UART Comm: Init >>Pixel Status: Pix Send On\nPixel Status: Pix Rec\nPixel Status: Update Pix Matrix>> UART Comm: Close" ("State(s) in Front (\"\")"), "State(s) in (\"\")"=w195) -> ("States Out"=w194:string)  [unwired: 13 in]
      }
      frame "Macro: Pixel Off" {
        n58 = call "addStatesToQueue.vi"("State(s) in Front (\"\")"="UART Comm: Init >>Pixel Status: Pix Send Off\nPixel Status: Pix Rec\nPixel Status: Update Pix Matrix>> UART Comm: Close" ("State(s) in Front (\"\")"), "State(s) in (\"\")"=w202) -> ("States Out"=w201:string)  [unwired: 13 in]
      }
      frame "Macro: All Pixel Check" {
        n59 = call "addStatesToQueue.vi"("State(s) in Front (\"\")"="UART Comm: Init >>All Pixel Status: Pix Send All\nAll Pixel Status: Pix Rec All" ("State(s) in Front (\"\")"), "State(s) in (\"\")"=w209) -> ("States Out"=w208:string)  [unwired: 13 in]
      }
      frame "Macro: Set Threshold" {
        n60 = call "addStatesToQueue.vi"("State(s) in Front (\"\")"="UART Comm: Init >>Threshold: Set Thresh\nThreshold: Get Thresh >> UART Comm: Close" ("State(s) in Front (\"\")"), "State(s) in (\"\")"=w216) -> ("States Out"=w215:string)  [unwired: 13 in]
      }
      frame "Macro: Set Clock" {
        n61 = call "addStatesToQueue.vi"("State(s) in Front (\"\")"="UART Comm: Init >>Clock: Set Clock\nClock: Get Clock>> UART Comm: Close" ("State(s) in Front (\"\")"), "State(s) in (\"\")"=w223) -> ("States Out"=w222:string)  [unwired: 13 in]
      }
      frame "Macro: Read Serial" {
        n62 = call "addStatesToQueue.vi"("State(s) in Front (\"\")"="UART Comm: Init >>Serial Number: Send Command\nSerial Number: Get Number\nSerial Number: Verify Number>>UART Comm: Close" ("State(s) in Front (\"\")"), "State(s) in (\"\")"=w230) -> ("States Out"=w229:string)  [unwired: 13 in]
      }
      frame "Macro: Update EEPROM" {
        n63 = call "addStatesToQueue.vi"("State(s) in Front (\"\")"="UART Comm: Init >>EEPROM: Update\nUART Comm: Close" ("State(s) in Front (\"\")"), "State(s) in (\"\")"=w237) -> ("States Out"=w236:string)  [unwired: 13 in]
      }
      frame "Macro: Reset EEPROM" {
        n64 = call "addStatesToQueue.vi"("State(s) in Front (\"\")"="UART Comm: Init >>EEPROM: Reset\nUART Comm: Close" ("State(s) in Front (\"\")"), "State(s) in (\"\")"=w244) -> ("States Out"=w243:string)  [unwired: 13 in]
      }
      frame "Macro: Exit" {
        # "Exit Macro\n(This is called once, when the VI exits)"
        n65 = Unbundle By Name(w253) -> ("Core.Close Panel on Exit?"=w252:bool)
        n66 = Select(t="UI: Front Panel State >> Close", s=w252, f="") -> (s? t:f=w249:string)
        n67 = call "addStatesToQueue.vi"("State(s) in (\"\")"=w249, "State(s) at Back (\"\")"="Data: Cleanup\nExit") -> ("States Out"=w247:string)  [unwired: 13 in]
        n68 = call "addStatesToQueue.vi"("State(s) in Front (\"\")"=w247, "State(s) in (\"\")"=w256) -> ("States Out"=w255:string)  [unwired: 13 in]
      }
      frame "---------- Core ----------" {
        # "Core Separator"
        n69 = call "addStatesToQueue.vi"("State(s) in (\"\")"=w262) -> ("States Out"=w261:string)  [unwired: 14 in]
      }
      frame Default {
        w274 = 42 items=["No error", "Argument error", "Memory is full", "Out of zone", "End of file", "File already open", "Generic file I/O error", "File not found", "File permission error", "Disk is full", "Duplicate path", "Too many files open", "System feature not enabled", "Resource file not found", "Cannot add resource", "Resource not found", "Image not found", "Image memory error", "Pen does not exist", "Config type invalid", "Config token not found", "Config parse error", "Config memory error", "Bad external code format", "Bad external code offset", "External code not present", "Null window", "Destroy window error", "Null menu", "Print aborted", "Bad print record", "Print driver error", "Windows error during printing", "Memory error during printing", "Print dialog error", "Generic print error", "Invalid device refnum", "Device not found", "Device parameter error", "Device unit error", "Cannot open device", "Device call aborted", "Generic error", "Cancelled by user", "Object ID too low", "Object ID too high", "Object not in heap", "Unknown heap", "Unknown object (invalid DefProc)", "Unknown object (DefProc not in table)", "Message out of range", "Invalid (null) method", "Unknown message", "Manager call not supported", "Bad address", "Network operation in progress", "Network operation timed out", "Connection is busy", "Network attribute not supported", "Network error", "Address in use", "System out of memory", "Connection aborted", "Connection refused", "Not connected", "Already connected", "Connection closed", "Initialization error (interapplication manager)", "Bad occurrence", "Wait on unbound occurrence handler", "Occurrence queue overflow", "Datalog type conflict", "Unused", "Unrecognized type (interapplication manager)", "Memory corrupt", "Failed to make temporary DLL", "Old CIN version", "Drag socket not found", "Failed to load drop-object", "Failed to register OLE object", "Failed to release OLE object", "Format specifier type mismatch", "Unknown format specifier", "Too few format specifiers", "Too many format specifiers", "Scan failed", "Newer CIN version", "Error converting to variant", "Runtime menu error", "Password tampered", "Variant attribute not found", "Incompatible variant data type", "Event data is not available", "Event Store is not present", "Occurrence is not found", "Event Queue is not created", "Event info is not available", "Refnum passed is NULL", "Error retrieving Class GUID", "Error retrieving CoClass GUID", "Error retrieving TypeLib GUID.", "Bad built application magic bytes.", "Specific driver is different from the specific driver associated with the Logical Name.", "There is no session opened to the class driver.", "Max Error", "MAX - Error with config objects", "MAX - Error loading configuration", "MAX - Group not supported"]
        # "Current State"
        # "Do not delete, rename, or modify this frame.\n(this is used to capture unhandled states and typos)"
        # "Handle mistyped state name (developer tool)"
        n70 = Format Into String(format string="Software Exception: Unhandled State \"%s\"." ("message"), error in=w270, w265) -> (resulting string=w273:string, error out=w272:errorcluster)  [unwired: 1 in]
        n71 = call <vilib>:"Error Cluster From Error Code.vi"("show call chain? (False)"=TRUE, "error in (no error)"=w272, "error message (\"\")"=w273, "error code (0)"=w274) -> ("error out"=w271:errorcluster)  [unwired: 5 in]
        n72 = call "addStatesToQueue.vi"("State(s) in (\"\")"=w269) -> ("States Out"=w268:string)  [unwired: 14 in]
      }
      frame "Initialize Core Data" {
        # "Do not delete, rename, or modify this frame.\n(this is used to determine panel behavior on exit)"
        # "originally closed?"
        # "exe?"
        # "If panel starts closed or is an EXE, then close it when we exit"
        n73 = property class="VI"() -> ("FP.State"=w280:T5)  [unwired: 2 in, 2 out]
        n74 = property class="App"() -> ("App.Kind"=w286:T6)  [unwired: 2 in, 2 out]
        n75 = control-ref of="Current VI Reference"() -> (w281:refnum<vi>)
        n76 = Equal?(x=w280, y=T5."Closed" ("Front Panel Window:State")) -> (x = y?=w278:bool)
        n77 = Equal?(x=w286, y=T6."Run Time System" ("Application:Kind")) -> (x = y?=w284:bool)
        n78 = Or(x=w278, y=w284) -> (x .or. y?=w282:bool)
        n79 = Bundle By Name(cluster=w283, "Core.Current VI Reference"=w281, "Core.Close Panel on Exit?"=w282) -> (w288:T9)
        n80 = call "addStatesToQueue.vi"("State(s) in (\"\")"=w290) -> ("States Out"=w289:string)  [unwired: 14 in]
      }
      frame "Error Handler" {
        # "Turn event mode off and close UART if error occured during event mode"
        # "Check what was going to be the next state"
        # "Close the UART communication if there was a timeout error"
        # "Unhandled Error -- Display it"
        # "Handle any errors here.\nYou can also output any states to clean-up after errors occur"
        # "Clear error"
        n81 = call "parseStateQueue.vi"("State Queue"=w302) -> ("Current State"=w300:string)  [unwired: 12 in, 2 out]
        n82 = Unbundle(w294) -> ("code"=w305:i32)  [unwired: 2 out]
        n83 = Equal?(x=-1073807339, y=w305) -> (x = y?=w304:bool)
        n84 = call <vilib>:"General Error Handler.vi"("error in (no error)"=w294) -> ()  [unwired: 10 in, 5 out]
        n85 = Equal?(x=w300, y="Event Mode: Rec Data") -> (x = y?=w298:bool)
        n86 = Equal?(x=w300, y="Event Mode: Close CSV") -> (x = y?=w297:bool)
        n87 = Select(t="UART Comm: Close", s=w304, f="") -> (s? t:f=w293:string)
        n88 = Or(x=w298, y=w297) -> (x .or. y?=w296:bool)
        n89 = Select(t="Event Mode: Close CSV >> Error!", s=w296, f=w293) -> (s? t:f=w292:string)
        n90 = call "addStatesToQueue.vi"("State(s) in Front (\"\")"=w292) -> ("States Out"=w311:string)  [unwired: 14 in]
      }
      frame "Exit" {
        # "Handles the exit funcitonality"
        n91 = call <vilib>:"Unset Busy.vi"("error in (no error)"=w314) -> ("error out"=w313:errorcluster)  [unwired: 10 in]
        n92 = call "addStatesToQueue.vi"("State(s) in (\"\")"=w319) -> ("States Out"=w318:string)  [unwired: 14 in]
      }
      frame "---------- Hardware ----------" {
        # "Hardware Separator"
        n93 = call "addStatesToQueue.vi"("State(s) in (\"\")"=w325) -> ("States Out"=w324:string)  [unwired: 14 in]
      }
      frame "Hardware: Setup DAQ" {
        # "Not used as of now"
        n94 = call "addStatesToQueue.vi"("State(s) in (\"\")"=w331) -> ("States Out"=w330:string)  [unwired: 14 in]
      }
      frame "---------- Data ----------" {
        n95 = call "addStatesToQueue.vi"("State(s) in (\"\")"=w337) -> ("States Out"=w336:string)  [unwired: 14 in]
      }
      frame "Data: Initialize" {
        w338 = T10 {"Pixel Number"=0, "Pixel En/Dis?"=FALSE, "Pixel Array"=[[TRUE, TRUE, TRUE, TRUE, TRUE, TRUE, TRUE, TRUE, TRUE, TRUE, TRUE, TRUE, TRUE, TRUE, TRUE, TRUE, TRUE], [TRUE, TRUE, TRUE, TRUE, TRUE, TRUE, TRUE, TRUE, TRUE, TRUE, TRUE, TRUE, TRUE, TRUE, TRUE, TRUE, TRUE], [TRUE, TRUE, TRUE, TRUE, TRUE, TRUE, TRUE, TRUE, TRUE, TRUE, TRUE, TRUE, TRUE, TRUE, TRUE, TRUE, TRUE], [TRUE, TRUE, TRUE, TRUE, TRUE, TRUE, TRUE, TRUE, TRUE, TRUE, TRUE, TRUE, TRUE, TRUE, TRUE, TRUE, TRUE], [TRUE, TRUE, TRUE, TRUE, TRUE, TRUE, TRUE, TRUE, TRUE, TRUE, TRUE, TRUE, TRUE, TRUE, TRUE, TRUE, TRUE], [TRUE, TRUE, TRUE, TRUE, TRUE, TRUE, TRUE, TRUE, TRUE, TRUE, TRUE, TRUE, TRUE, TRUE, TRUE, TRUE, TRUE], [TRUE, TRUE, TRUE, TRUE, TRUE, TRUE, TRUE, TRUE, TRUE, TRUE, TRUE, TRUE, TRUE, TRUE, TRUE, TRUE, TRUE], [TRUE, TRUE, TRUE, TRUE, TRUE, TRUE, TRUE, TRUE, TRUE, TRUE, TRUE, TRUE, TRUE, TRUE, TRUE, TRUE, TRUE], [TRUE, TRUE, TRUE, TRUE, TRUE, TRUE, TRUE, TRUE, TRUE, TRUE, TRUE, TRUE, TRUE, TRUE, TRUE, TRUE, TRUE], [TRUE, TRUE, TRUE, TRUE, TRUE, TRUE, TRUE, TRUE, TRUE, TRUE, TRUE, TRUE, TRUE, TRUE, TRUE, TRUE, TRUE], [TRUE, TRUE, TRUE, TRUE, TRUE, TRUE, TRUE, TRUE, TRUE, TRUE, TRUE, TRUE, TRUE, TRUE, TRUE, TRUE, TRUE], [TRUE, TRUE, TRUE, TRUE, TRUE, TRUE, TRUE, TRUE, TRUE, TRUE, TRUE, TRUE, TRUE, TRUE, TRUE, TRUE, TRUE], [TRUE, TRUE, TRUE, TRUE, TRUE, TRUE, TRUE, TRUE, TRUE, TRUE, TRUE, TRUE, TRUE, TRUE, TRUE, TRUE, TRUE], [TRUE, TRUE, TRUE, TRUE, TRUE, TRUE, TRUE, TRUE, TRUE, TRUE, TRUE, TRUE, TRUE, TRUE, TRUE, TRUE, TRUE], [TRUE, TRUE, TRUE, TRUE, TRUE, TRUE, TRUE, TRUE, TRUE, TRUE, TRUE, TRUE, TRUE, TRUE, TRUE, TRUE, TRUE], [TRUE, TRUE, TRUE, TRUE, TRUE, TRUE, TRUE, TRUE, TRUE, TRUE, TRUE, TRUE, TRUE, TRUE, TRUE, TRUE, TRUE]], "Disabled Pixels"=[]}  # Pixel Status 2
        w339 = T10 {"Pixel Number"=0, "Pixel En/Dis?"=FALSE, "Pixel Array"=[[TRUE, TRUE, TRUE, TRUE, TRUE, TRUE, TRUE, TRUE, TRUE, TRUE, TRUE, TRUE, TRUE, TRUE, TRUE, TRUE, TRUE], [TRUE, TRUE, TRUE, TRUE, TRUE, TRUE, TRUE, TRUE, TRUE, TRUE, TRUE, TRUE, TRUE, TRUE, TRUE, TRUE, TRUE], [TRUE, TRUE, TRUE, TRUE, TRUE, TRUE, TRUE, TRUE, TRUE, TRUE, TRUE, TRUE, TRUE, TRUE, TRUE, TRUE, TRUE], [TRUE, TRUE, TRUE, TRUE, TRUE, TRUE, TRUE, TRUE, TRUE, TRUE, TRUE, TRUE, TRUE, TRUE, TRUE, TRUE, TRUE], [TRUE, TRUE, TRUE, TRUE, TRUE, TRUE, TRUE, TRUE, TRUE, TRUE, TRUE, TRUE, TRUE, TRUE, TRUE, TRUE, TRUE], [TRUE, TRUE, TRUE, TRUE, TRUE, TRUE, TRUE, TRUE, TRUE, TRUE, TRUE, TRUE, TRUE, TRUE, TRUE, TRUE, TRUE], [TRUE, TRUE, TRUE, TRUE, TRUE, TRUE, TRUE, TRUE, TRUE, TRUE, TRUE, TRUE, TRUE, TRUE, TRUE, TRUE, TRUE], [TRUE, TRUE, TRUE, TRUE, TRUE, TRUE, TRUE, TRUE, TRUE, TRUE, TRUE, TRUE, TRUE, TRUE, TRUE, TRUE, TRUE], [TRUE, TRUE, TRUE, TRUE, TRUE, TRUE, TRUE, TRUE, TRUE, TRUE, TRUE, TRUE, TRUE, TRUE, TRUE, TRUE, TRUE], [TRUE, TRUE, TRUE, TRUE, TRUE, TRUE, TRUE, TRUE, TRUE, TRUE, TRUE, TRUE, TRUE, TRUE, TRUE, TRUE, TRUE], [TRUE, TRUE, TRUE, TRUE, TRUE, TRUE, TRUE, TRUE, TRUE, TRUE, TRUE, TRUE, TRUE, TRUE, TRUE, TRUE, TRUE], [TRUE, TRUE, TRUE, TRUE, TRUE, TRUE, TRUE, TRUE, TRUE, TRUE, TRUE, TRUE, TRUE, TRUE, TRUE, TRUE, TRUE], [TRUE, TRUE, TRUE, TRUE, TRUE, TRUE, TRUE, TRUE, TRUE, TRUE, TRUE, TRUE, TRUE, TRUE, TRUE, TRUE, TRUE], [TRUE, TRUE, TRUE, TRUE, TRUE, TRUE, TRUE, TRUE, TRUE, TRUE, TRUE, TRUE, TRUE, TRUE, TRUE, TRUE, TRUE], [TRUE, TRUE, TRUE, TRUE, TRUE, TRUE, TRUE, TRUE, TRUE, TRUE, TRUE, TRUE, TRUE, TRUE, TRUE, TRUE, TRUE], [TRUE, TRUE, TRUE, TRUE, TRUE, TRUE, TRUE, TRUE, TRUE, TRUE, TRUE, TRUE, TRUE, TRUE, TRUE, TRUE, TRUE]], "Disabled Pixels"=[]}  # Pixel Status 1
        w341 = T11 {"User Name"="", "Short Description"="", "Description"="", "CZT Threshold 1"=0, "CZT Threshold 2"=0}  # User & Config Data
        w342 = T12 {"Dump txt file path"=path "", "Data Buffer"="", "Valid Data in Buffer"=0, "CSV file path"=path "", "Fits File name"="", "Test Start time"=timestamp(0 s since 1904-01-01)}  # CSV File Data
        w344 = T13 {"Current VI Reference"=refnum, "Close Panel on Exit?"=FALSE}  # Core
        w343 = u32 0  # Iteration Count
        w346 = 0.0  # Start Time
        w347 = 0.0  # Acquisition Period
        w348 = TRUE  # Stop Pressed?
        # "do not delete - used by framework"
        # "Data names and types of shift register data are defined by this bundle."
        # "Initialize the shift-register data, here.\n(data names are defined by what you wire into the bundle function)"
        n96 = Bundle("Core"=w344, "Stop Pressed?"=w348, "Start Time"=w346, "Acquisition Period"=w347, "Iteration Count"=w343, "CSV File Data"=w342, "User & Config Data"=w341, "Pixel Status 1"=w339, "Pixel Status 2"=w338) -> (w350:T9)  [unwired: 1 in]
        n97 = call "addStatesToQueue.vi"("State(s) in (\"\")"=w352) -> ("States Out"=w351:string)  [unwired: 14 in]
      }
      frame "Data: Cleanup" {
        # "Cleanup any data and references, here.\n(this is called automatically, by the Macro: Exit)"
        n98 = Unbundle By Name(w355) -> ("Core.Current VI Reference"=w358:refnum<vi>)
        n99 = Close Reference(reference=w358, error in (no error)=w357) -> (error out=w356:errorcluster)
        n100 = call "addStatesToQueue.vi"("State(s) in (\"\")"=w360) -> ("States Out"=w359:string)  [unwired: 14 in]
      }
      frame "---------- UI ----------" {
        # "UI Separator"
        n101 = call "addStatesToQueue.vi"("State(s) in (\"\")"=w366) -> ("States Out"=w365:string)  [unwired: 14 in]
      }
      frame "UI: Initialize" {
        w381 = T7."Disabled and Grayed Out" ("Disabled")
        # "Initialize the User Interface, here.\n(this is called automatically, by the Macro: Init)"
        n102 = invoke on="Test Description" class="Str" method="Reinit To Default"(error in=w373) -> (error out=w392:errorcluster)  [unwired: 2 in, 2 out]
        n103 = invoke on="Select Threshold Value" class="Slide (strict)" method="Reinit To Default"(error in=w373) -> (error out=w393:errorcluster)  [unwired: 2 in, 2 out]
        n104 = invoke on="CZT 1 Thresh" class="DigNum (strict)" method="Reinit To Default"(error in=w373) -> (error out=w394:errorcluster)  [unwired: 2 in, 2 out]
        n105 = invoke on="CZT 1 Serial In" class="DigNum (strict)" method="Reinit To Default"(error in=w373) -> (error out=w375:errorcluster)  [unwired: 2 in, 2 out]
        n106 = invoke on="CZT 1 Serial" class="DigNum (strict)" method="Reinit To Default"(error in=w373) -> (error out=w391:errorcluster)  [unwired: 2 in, 2 out]
        n107 = invoke on="CZT 2 Thresh" class="DigNum (strict)" method="Reinit To Default"(error in=w373) -> (error out=w390:errorcluster)  [unwired: 2 in, 2 out]
        n108 = invoke on="Column" class="DigNum (strict)" method="Reinit To Default"(error in=w391) -> (error out=w396:errorcluster)  [unwired: 2 in, 2 out]
        n109 = invoke on="Row" class="Str" method="Reinit To Default"(error in=w373) -> (error out=w397:errorcluster)  [unwired: 2 in, 2 out]
        n110 = invoke on="Pixel Matrix Status" class="Arr (strict)" method="Reinit To Default"(error in=w390) -> (error out=w398:errorcluster)  [unwired: 2 in, 2 out]
        n111 = invoke on="Event Mode" class="Bool (strict)" method="Reinit To Default"(error in=w392) -> (error out=w400:errorcluster)  [unwired: 2 in, 2 out]
        n112 = invoke on="User Name" class="Str" method="Reinit To Default"(error in=w393) -> (error out=w401:errorcluster)  [unwired: 2 in, 2 out]
        n113 = invoke on="Short Description" class="Str" method="Reinit To Default"(error in=w394) -> (error out=w395:errorcluster)  [unwired: 2 in, 2 out]
        n114 = invoke on="CZT 2 Serial In" class="DigNum (strict)" method="Reinit To Default"(error in=w375) -> (error out=w374:errorcluster)  [unwired: 2 in, 2 out]
        n115 = invoke on="Choose Pixel" class="DigNum (strict)" method="Reinit To Default"(error in=w396) -> (error out=w389:errorcluster)  [unwired: 2 in, 2 out]
        n116 = property on="Stop" class="Bool (strict)"(error in=w397, "DisabledEnum"=w381) -> (error out=w383:errorcluster)  [unwired: 1 in, 1 out]
        n117 = invoke on="FITS File" class="Bool (strict)" method="Reinit To Default"(error in=w398) -> (error out=w385:errorcluster)  [unwired: 2 in, 2 out]
        n118 = invoke on="Events Count" class="DigNum (strict)" method="Reinit To Default"(error in=w400) -> (error out=w386:errorcluster)  [unwired: 2 in, 2 out]
        n119 = invoke on="Time elapsed" class="DigNum (strict)" method="Reinit To Default"(error in=w401) -> (error out=w368:errorcluster)  [unwired: 2 in, 2 out]
        n120 = invoke on="Acquisition Period" class="Clust (strict)" method="Reinit To Default"(error in=w395) -> (error out=w370:errorcluster)  [unwired: 2 in, 2 out]
        n121 = invoke on="Serial1 Same?" class="Bool (strict)" method="Reinit To Default"(error in=w374) -> (error out=w376:errorcluster)  [unwired: 2 in, 2 out]
        n122 = property on="Open CSV" class="Bool"(error in=w383, "DisabledEnum"=w381) -> (error out=w382:errorcluster)  [unwired: 1 in, 1 out]
        n123 = invoke on="Pixel Status 2" class="Arr (strict)" method="Reinit To Default"(error in=w370) -> (error out=w369:errorcluster)  [unwired: 2 in, 2 out]
        n124 = invoke on="CZT 1 Frequency" class="DigNum (strict)" method="Reinit To Default"(error in=w385) -> (error out=w380:errorcluster)  [unwired: 2 in, 2 out]
        n125 = invoke on="Pixel Status 1" class="Arr (strict)" method="Reinit To Default"(error in=w368) -> (error out=w367:errorcluster)  [unwired: 2 in, 2 out]
        n126 = invoke on="Serial2 Same?" class="Bool (strict)" method="Reinit To Default"(error in=w376) -> (error out=w372:errorcluster)  [unwired: 2 in, 2 out]
        n127 = invoke on="CZT 2 Serial" class="DigNum (strict)" method="Reinit To Default"(error in=w389) -> (error out=w371:errorcluster)  [unwired: 2 in, 2 out]
        n128 = invoke on="CZT 2 Frequency" class="DigNum (strict)" method="Reinit To Default"(error in=w386) -> (error out=w388:errorcluster)  [unwired: 2 in, 2 out]
        n129 = invoke on="Set Clock" class="Bool" method="Reinit To Default"(error in=w382) -> (error out=w387:errorcluster)  [unwired: 2 in, 2 out]
        n130 = invoke on="Noisy Pixel List" class="Arr (strict)" method="Reinit To Default"(error in=w380) -> (error out=w379:errorcluster)  [unwired: 2 in, 2 out]
        n131 = property on="Start Event" class="Bool"(error in=w367, "Key Focus"=TRUE) -> (error out=w377:errorcluster)  [unwired: 1 in, 1 out]
        n132 = Merge Errors(w371, w387, w379, w388, w377, w369, w372) -> (w384:errorcluster)
        n133 = call "addStatesToQueue.vi"("State(s) in (\"\")"=w405) -> ("States Out"=w404:string)  [unwired: 14 in]
      }
      frame "UI: Cursor Set" {
        # "Argument"
        # "Set and Unset Cursor Busy.\n(Usage: \"UI: Cursor Set >> Busy|Idle\")"
        n134 = case shown="\"Idle\", Default" w408 {
          tunnel: w410 -> [w415 w417]
          tunnel: [w414 w416] -> w409
          frame "Idle", Default {
            n135 = call <vilib>:"Unset Busy.vi"("error in (no error)"=w415) -> ("error out"=w414:errorcluster)  [unwired: 10 in]
          }
          frame "Busy" {
            n136 = call <vilib>:"Set Busy.vi"("error in (no error)"=w417) -> ("error out"=w416:errorcluster)  [unwired: 9 in, 1 out]
          }
        }
        n137 = call "addStatesToQueue.vi"("State(s) in (\"\")"=w413) -> ("States Out"=w412:string)  [unwired: 14 in]
      }
      frame "UI: Front Panel State" {
        # "Argument"
        # "Set Front Panel Open or Closed\n(Usage: \"UI: Front Panel State >> Open|Close\")"
        n138 = Unbundle By Name(w422) -> ("Core.Current VI Reference"=w421:refnum<vi>)
        n139 = case shown="\"Open\", \"Standard\", Default" w420 {
          tunnel: w424 -> [w432 w447 w458 w471 w484]
          tunnel: [w434 w448 w460 w473 w486] -> w423
          tunnel: w421 -> [w433 w445 w459 w472 w485]
          frame "Open", "Standard", Default {
            w427 = T5."Standard" ("State")
            n140 = property class="VI"(reference=w433, error in=w432) -> (reference out=w430:refnum<vi>, error out=w431:errorcluster, "FP.State"=w429:T5)
            n141 = Not Equal?(x=w429, y=w427) -> (x != y?=w428:bool)
            n142 = case shown="True" w428 {
              tunnel: [w438 w440] -> w434
              tunnel: w431 -> [w437 w440]
              tunnel: w430 -> [w436 _]
              tunnel: w427 -> [w435 _]
              frame True {
                n143 = invoke class="VI" method="FP.Open"(reference=w436, error in=w437, "Activate"=FALSE, "State"=w435) -> (error out=w438:errorcluster)  [unwired: 1 in, 4 out]
              }
              frame False {
              }
            }
          }
          frame "Close", "Closed" {
            n144 = property class="VI"(reference=w445, error in=w447) -> (reference out=w444:refnum<vi>, error out=w446:errorcluster, "FP.State"=w442:T5)
            n145 = Not Equal?(x=w442, y=T5."Closed" ("Front Panel Window:State")) -> (x != y?=w441:bool)
            n146 = case shown="True" w441 {
              tunnel: [w449 w452] -> w448
              tunnel: w446 -> [w449 w451]
              tunnel: w444 -> [_ w450]
              frame False {
              }
              frame True {
                n147 = invoke class="VI" method="FP.Close"(reference=w450, error in=w451) -> (error out=w452:errorcluster)  [unwired: 1 in, 2 out]
              }
            }
          }
          frame "Hidden", "Hide" {
            w453 = T5."Hidden" ("State")
            n148 = property class="VI"(reference=w459, error in=w458) -> (reference out=w456:refnum<vi>, error out=w457:errorcluster, "FP.State"=w455:T5)
            n149 = Not Equal?(x=w455, y=w453) -> (x != y?=w454:bool)
            n150 = case shown="True" w454 {
              tunnel: [w464 w465] -> w460
              tunnel: w457 -> [w463 w465]
              tunnel: w456 -> [w462 _]
              tunnel: w453 -> [w461 _]
              frame True {
                n151 = invoke class="VI" method="FP.Open"(reference=w462, error in=w463, "State"=w461) -> (error out=w464:errorcluster)  [unwired: 2 in, 4 out]
              }
              frame False {
              }
            }
          }
          frame "Minimize", "Minimized" {
            w466 = T5."Minimized" ("State")
            n152 = property class="VI"(reference=w472, error in=w471) -> (reference out=w469:refnum<vi>, error out=w470:errorcluster, "FP.State"=w468:T5)
            n153 = Not Equal?(x=w468, y=w466) -> (x != y?=w467:bool)
            n154 = case shown="True" w467 {
              tunnel: [w477 w478] -> w473
              tunnel: w470 -> [w476 w478]
              tunnel: w469 -> [w475 _]
              tunnel: w466 -> [w474 _]
              frame True {
                n155 = invoke class="VI" method="FP.Open"(reference=w475, error in=w476, "State"=w474) -> (error out=w477:errorcluster)  [unwired: 2 in, 4 out]
              }
              frame False {
              }
            }
          }
          frame "Maximize", "Maximized" {
            w479 = T5."Maximized" ("State")
            n156 = property class="VI"(reference=w485, error in=w484) -> (reference out=w482:refnum<vi>, error out=w483:errorcluster, "FP.State"=w481:T5)
            n157 = Not Equal?(x=w481, y=w479) -> (x != y?=w480:bool)
            n158 = case shown="True" w480 {
              tunnel: [w490 w491] -> w486
              tunnel: w483 -> [w489 w491]
              tunnel: w482 -> [w488 _]
              tunnel: w479 -> [w487 _]
              frame True {
                n159 = invoke class="VI" method="FP.Open"(reference=w488, error in=w489, "State"=w487) -> (error out=w490:errorcluster)  [unwired: 2 in, 4 out]
              }
              frame False {
              }
            }
          }
        }
        n160 = call "addStatesToQueue.vi"("State(s) in (\"\")"=w426) -> ("States Out"=w425:string)  [unwired: 14 in]
      }
      frame "---------- Event Mode ----------" {
        # "Event Mode Separator"
        n161 = call "addStatesToQueue.vi"("State(s) in (\"\")"=w497) -> ("States Out"=w496:string)  [unwired: 14 in]
      }
      frame "Event Mode: Data Init" {
        w508 = FALSE  # Stop Pressed?
        w506 = u32 0  # Iteration Count
        w511 = path ""  # Dump txt file path
        w507 = 0.0  # Start Time
        # "Initialize the data to be used in the event mode"
        n162 = invoke on="FITS File" class="Bool (strict)" method="Reinit To Default"(error in=w503) -> (error out=w502:errorcluster)  [unwired: 2 in, 2 out]
        n163 = invoke on="Events Count" class="DigNum (strict)" method="Reinit To Default"(error in=w502) -> (error out=w501:errorcluster)  [unwired: 2 in, 2 out]
        n164 = call "csvHeaderGen.vi"() -> ("Valid Data in Buffer"=w510:i32, "Data Buffer"=w509:string)  [unwired: 10 in]
        n165 = Bundle By Name(cluster=w505, "Stop Pressed?"=w508, "Start Time"=w507, "Iteration Count"=w506, "CSV File Data.Dump txt file path"=w511, "CSV File Data.Data Buffer"=w509, "CSV File Data.Valid Data in Buffer"=w510) -> (w504:T9)
        n166 = invoke on="Time elapsed" class="DigNum (strict)" method="Reinit To Default"(error in=w501) -> (error out=w498:errorcluster)  [unwired: 2 in, 2 out]
        n167 = invoke on="Event Mode" class="Bool (strict)" method="Reinit To Default"(error in=w498) -> (error out=w500:errorcluster)  [unwired: 2 in, 2 out]
        n168 = call "addStatesToQueue.vi"("State(s) in (\"\")"=w514) -> ("States Out"=w513:string)  [unwired: 14 in]
      }
      frame "Event Mode: Data Get" {
        # "Template Separator\n(You can make a copy of, or modify, this frame)"
        n169 = property on="CZT 1 Thresh" class="DigNum (strict)"(error in=w518) -> (error out=w517:errorcluster, "Value"=w515:u16)  [unwired: 1 in, 1 out]
        n170 = Unbundle("Acquisition Period") -> ("Hours"=w525:u32, "Minutes"=w532:u32, "Seconds"=w530:u32)
        n171 = expression code="x*3600"(w525) -> (w526:u32)
        n172 = expression code="x*60"(w532) -> (w531:u32)
        n173 = property on="CZT 2 Thresh" class="DigNum (strict)"(error in=w517) -> (error out=w521:errorcluster, "Value"=w516:u16)  [unwired: 1 in, 1 out]
        n174 = Compound Arithmetic op=ADD(w526, w531, w530) -> (w529:u32)
        n175 = Bundle("User Name"="User Name", "Short Description"="Short Description", "Test Description"="Test Description", "Value"=w515, "Value"=w516) -> (w520:T14)  [unwired: 1 in]
        n176 = Bundle By Name(cluster=w524, "Acquisition Period"=w529, "User & Config Data"=w520) -> (w523:T9)
        n177 = call "addStatesToQueue.vi"("State(s) in (\"\")"=w536) -> ("States Out"=w535:string)  [unwired: 14 in]
      }
      frame "Event Mode: Data Verif" {
        # "Checks if all the required data has been entered by the user! If all okay them moves to next state as per macro."
        # "Verify the data entered by the user if it is within its limits"
        n178 = Unbundle By Name(w550) -> ("User & Config Data.Description"=w542:string, "Acquisition Period"=w548:dbl, "User & Config Data.User Name"=w547:string, "User & Config Data.Short Description"=w546:string, "User & Config Data.CZT Threshold 1"=w545:u16)  [unwired: 1 out]
        n179 = call "chkEvntSet.vi"("Description"=w542, "Acquisition Period"=w548, "error in (no error)"=w551, "Current Threshold Value"=w545, "Short Description"=w546, "User Name"=w547) -> ("error out"=w540:errorcluster)  [unwired: 5 in]
        n180 = Select(t="", s=w540, f=w544) -> (s? t:f=w537:string)
        n181 = property on="Stop" class="Bool (strict)"(error in=w540, "DisabledEnum"=T7."Enabled" ("Disabled")) -> (error out=w539:errorcluster)  [unwired: 1 in, 1 out]
        n182 = call "addStatesToQueue.vi"("State(s) in (\"\")"=w537) -> ("States Out"=w552:string)  [unwired: 14 in]
      }
      frame "Event Mode: Send Cmd" {
        # "Send the Event mode start command and start recieving the code"
        n183 = property on="Stop" class="Bool (strict)"(error in=w555) -> (error out=w554:errorcluster, "Value"=w553:bool)  [unwired: 1 in, 1 out]
        n184 = case shown="True" w553 {
          selector: w553 -> [_ w594]
          tunnel: w562 -> [w591 w599]
          tunnel: [w590 w599] -> w561
          tunnel: w554 -> [w568 w596]
          tunnel: [w587 w593] -> w560
          tunnel: [w586 "Event Mode: Close CSV"] -> w559
          tunnel: [w576 _] -> w558
          tunnel: w557 -> [w577 w592]
          tunnel: [w566 w595] -> w556
          frame False {
            # "Generate the dump file name and create storage directory"
            # "If there is no error log current timer value"
            n185 = Unbundle(w577) -> ("Acquisition Period"=w569:dbl, "CSV File Data"=w582:T12, "User & Config Data"=w580:T11)  [unwired: 6 out]
            n186 = Unbundle(w580) -> ("User Name"=w572:string, "Short Description"=w571:string, "CZT Threshold 1"=w570:u16)  [unwired: 2 out]
            n187 = Get Date/Time In Seconds() -> (seconds since 1Jan1904=w573:timestamp)
            n188 = call "csvNameGenerate.vi"("User Name"=w572, "time stamp"=w573, "Short Description"=w571, "Threshold Value"=w570, "Acquisition Period"=w569, "error in"=w568) -> ("Dump file path"=w574:path, "Byte Stream File out"=w576:refnum<file>, "File Name"=w575:string, "error out"=w567:errorcluster)  [unwired: 6 in]
            n189 = Bundle(cluster=w582, "Dump txt file path"=w574, "Fits File name"=w575, "Test Start time"=w573) -> (w581:T12)  [unwired: 3 in]
            n190 = VISA Write(VISA resource name=w591, write buffer=" ÿU" ("Event mode ON w/o Emulator"), error in (no error)=w567) -> (VISA resource name out=w590:refnum<visa-resource-name>, return count=w579:u32, error out=w566:errorcluster)
            n191 = Greater Than 0?(x=w579) -> (x > 0?=→"Event Mode":bool)
            n192 = call <vilib>:"High Resolution Relative Seconds.vi"() -> ("relative seconds"=w585:dbl)
            n193 = Select(t=0.0, s=w566, f=w585) -> (s? t:f=w584:dbl)
            n194 = Select(t="", s=w566, f="Event Mode: Rec Data") -> (s? t:f=w586:string)
            n195 = Bundle(cluster=w577, "Start Time"=w584, "CSV File Data"=w581) -> (w587:T9)  [unwired: 7 in]
          }
          frame True {
            n196 = Bundle By Name(cluster=w592, "Stop Pressed?"=w594) -> (w593:T9)
            n197 = property on="Stop" class="Bool (strict)"(error in=w596, "Value"=FALSE ("Stop")) -> (error out=w595:errorcluster)  [unwired: 1 in, 1 out]
          }
        }
        n198 = call "addStatesToQueue.vi"("State(s) in Front (\"\")"=w559, "State(s) in (\"\")"=w564) -> ("States Out"=w563:string)  [unwired: 13 in]
      }
      frame "Event Mode: Rec Data" {
        # "Check if the stop button is pressed, each loop"
        # "Record the event mode data into a csv file"
        n199 = case shown="False" "Stop" {
          selector: "Stop" -> [_ w654]
          tunnel: [w642 "Event Mode: Close CSV"] -> w609
          tunnel: w608 -> [w641 w659]
          tunnel: w607 -> [w640 w657]
          tunnel: [w639 w659] -> w606
          tunnel: [w617 w655] -> w605
          tunnel: w604 -> [w637 w660]
          tunnel: [w636 w660] -> w603
          tunnel: [w624 w652] -> w602
          tunnel: w601 -> [w635 w653]
          frame False {
            # "Writes formatted data to the dump txt file"
            # "Formats input data as per csv"
            # "Elapsed time generation & comparison logic"
            n200 = Unbundle(w635) -> ("Start Time"=w647:dbl, "Acquisition Period"=w645:dbl, "Iteration Count"=w613:u32, "CSV File Data"=w632:T12)  [unwired: 5 out]
            n201 = call <vilib>:"High Resolution Relative Seconds.vi"() -> ("relative seconds"=w646:dbl)
            n202 = VISA Read(VISA resource name=w641, byte count=u32 50, error in (no error)=w640) -> (VISA resource name out=w639:refnum<visa-resource-name>, read buffer=w621:string, error out=w615:errorcluster)  [unwired: 1 out]
            n203 = Subtract(x=w646, y=w647) -> (x-y=w638:dbl)
            "Time elapsed" <- w638
            n204 = Less?(x=w638, y=w645) -> (x < y?=w620:bool)
            n205 = Increment(x=w613) -> (x+1=w614:u32)
            n206 = Select(t=w613, s=w615, f=w614) -> (s? t:f=w612:u32)
            "Events Count" <- w612
            n207 = call "csvFormatter.vi"("Iteration"=w612, "error in (no error)"=w615, "Sensor Data In"=w621) -> ("error out"=w634:errorcluster, "CSV formatted String"=w633:string)  [unwired: 7 in]
            n208 = Unbundle(w632) -> ("Dump txt file path"=w629:path, "Data Buffer"=w630:string, "Valid Data in Buffer"=w631:i32, "CSV file path"=w625:path, "Fits File name"=w623:string, "Test Start time"=w622:timestamp)
            n209 = call "csvBitWrite.vi"("data buffer"=w630, "valid data in buffer"=w631, "error in (no error)"=w634, "CSV Formatted String"=w633, "Byte Stream File in"=w637) -> ("error out"=w618:errorcluster, "Valid Data Buf OUT"=w627:i32, "Data buffer OUT"=w628:string, "Byte Stream File out"=w636:refnum<file>)  [unwired: 3 in]
            n210 = Bundle("Dump txt file path"=w629, "Data buffer OUT"=w628, "Valid Data Buf OUT"=w627, "CSV file path"=w625, "Fits File name"=w623, "Test Start time"=w622) -> (w626:T15)  [unwired: 1 in]
            n211 = Bundle(cluster=w635, "Iteration Count"=w612, "CSV File Data"=w626) -> (w624:T9)  [unwired: 7 in]
            n212 = disable-structure shown="Disabled" {
              disable-tunnel: _ -> [w649 _]
              disable-tunnel: [w648 TRUE] -> _
              frame Disabled {
                n213 = Less?(x=w649, y="Iteration Limit") -> (x < y?=w648:bool)
              }
              frame Enabled {
              }
            }
            n214 = call <vilib>:"Clear Errors.vi"("error in (no error)"=w618, "specific error code to clear (0: all)"=-1073807339) -> ("error out"=w617:errorcluster)  [unwired: 4 in, 1 out]
            n215 = Select(t="Event Mode: Rec Data", s=w620, f="Event Mode: Close CSV") -> (s? t:f=w642:string)
          }
          frame True {
            # "Latched button resetted"
            # "Stop button Pressed; End data acquisition"
            n216 = Bundle By Name(cluster=w653, "Stop Pressed?"=w654) -> (w652:T9)
            n217 = property on="Stop" class="Bool (strict)"(error in=w657, "Value"=FALSE ("Stop")) -> (error out=w655:errorcluster)  [unwired: 1 in, 1 out]
          }
        }
        n218 = call "addStatesToQueue.vi"("State(s) in Front (\"\")"=w609, "State(s) in (\"\")"=w611) -> ("States Out"=w610:string)  [unwired: 13 in]
      }
      frame "Event Mode: Close CSV" {
        w663 = " \u0000U"  # Event mode OFF
        # "Changes dump file extension to csv"
        # "Close file ref"
        # "Write last line of data"
        # "Close the reference to the CSV file and change the extension from .txt to .csv"
        n219 = Unbundle(w682) -> ("CSV File Data"=w678:T12)  [unwired: 8 out]
        n220 = Unbundle(w678) -> ("Data Buffer"=w680:string, "Valid Data in Buffer"=w679:i32)  [unwired: 4 out]
        n221 = String Subset(string=w680, length (rest)=w679) -> (substring=w689:string)  [unwired: 1 in]
        n222 = VISA Write(VISA resource name=w675, write buffer=w663, error in (no error)=w674) -> (VISA resource name out=w673:refnum<visa-resource-name>, error out=w668:errorcluster)  [unwired: 1 out]
        n223 = Write to Text File(file (use dialog)=w688, text=w689, error in=w674) -> (refnum out=w686:refnum<file>, error out=w687:errorcluster)  [unwired: 1 in, 1 out]
        n224 = Close File(refnum=w686, error in=w687) -> (path=w670:path, error out=w685:errorcluster)
        n225 = call "changeEXT.vi"("Path"=w670, "error in (no error)"=w685, "New Extension"="csv") -> ("error out"=w672:errorcluster, "Success?"=w669:bool, "Out CSV Path"=w677:path)  [unwired: 6 in]
        n226 = Bundle(cluster=w678, "CSV file path"=w677) -> (w676:T12)  [unwired: 5 in]
        n227 = Equal?(x=w666, y="Error!") -> ()  [unwired: 1 out]
        n228 = Bundle(cluster=w682, "CSV File Data"=w676) -> (w681:T9)  [unwired: 8 in]
        n229 = Select(t="Event Mode: Make FITS", s=w669, f="") -> (s? t:f=w661:string)
        n230 = invoke on="Event Mode" class="Bool (strict)" method="Reinit To Default"(error in=w668) -> (error out=w667:errorcluster)  [unwired: 2 in, 2 out]
        n231 = disable-structure shown="Enabled" {
          disable-tunnel: [w693 w695] -> w664
          disable-tunnel: w661 -> [w692 w695]
          frame Disabled {
            n232 = Select(t="Event Mode: Update Graphs", f=w692) -> (s? t:f=w693:string)  [unwired: 1 in]
          }
          frame Enabled {
          }
        }
        n233 = Merge Errors(w667, w672) -> (w671:errorcluster)
        n234 = call "addStatesToQueue.vi"("State(s) in Front (\"\")"=w664, "State(s) in (\"\")"=w691) -> ("States Out"=w690:string)  [unwired: 13 in]
      }
      frame "Event Mode: Make FITS" {
        # "FITS Metadata Requirement:\n>File name // Str- Done\n>Date Time //Str -done\n>User Name //Str - Done\n>Comments //Str - done\n>Original File Path //Str-done\n>Threshold Value //Int-done\n>Pixel data //Str-done\n>Acquisition Period //Str-done\n>CZT Serial Number //Str - not started"
        # "Calls a python function to convert the .csv file to a .fits file"
        n235 = Unbundle By Name(w696) -> ("CSV File Data.Fits File name"=w707:string, "User & Config Data.User Name"=w710:string, "User & Config Data.Short Description"=w709:string, "User & Config Data.Description"=w703:string, "CSV File Data.Test Start time"=w704:timestamp, "Acquisition Period"=w708:dbl, "User & Config Data.CZT Threshold 1"=w705:u16, "Pixel Status 1.Disabled Pixels"=w706:u8[])  [unwired: 1 out]
        n236 = property on="Stop" class="Bool (strict)"(error in=w701, "DisabledEnum"=T7."Disabled and Grayed Out" ("Disabled")) -> (error out=w700:errorcluster)  [unwired: 1 in, 1 out]
        n237 = Bundle("Fits File name"=w707, "User Name"=w710, "Short Description"=w709, "Description"=w703, "Test Start time"=w704, "Acquisition Period"=w708, "CZT Threshold 1"=w705, "Disabled Pixels"=w706) -> ()  [unwired: 1 in, 1 out]
        n238 = property on="Open CSV" class="Bool"(error in=w700, "DisabledEnum"=T7."Enabled" ("Disabled")) -> (error out=w698:errorcluster)  [unwired: 1 in, 1 out]
        n239 = call "addStatesToQueue.vi"("State(s) in Front (\"\")"="Event Mode: Update Graphs", "State(s) in (\"\")"=w697) -> ("States Out"=w714:string)  [unwired: 13 in]
      }
      frame "Event Mode: Update Graphs" {
        # "Display the channel graphs"
        # "Calculate and display the energy spectrum"
        # "Clean CSV of garbage data (if any)"
        # "Reads the event data and updates the graphs"
        n240 = Unbundle By Name(w729) -> ("CSV File Data.CSV file path"=w728:path)
        n241 = call "csvCleaner.vi"("error in (no error)"=w727, "CSV Input File"=w728) -> ("error out"=w718:errorcluster, "Clean No Dups Size"=→"Clean No Dups Size":i32[], "all rows"=w715:string[][], "Input Size"=→"Input Size":i32[])  [unwired: 2 in, 4 out]
        "All rows" <- w715
        n242 = call "energyGraph.vi"("error in (no error)"=w718, "Clean+No Dups"=w715) -> ("error out"=w717:errorcluster, "Clean+No Dups Out"=w716:string[][], "Histogram Graph"=→"Energy Spectrum":T2)  [unwired: 7 in]
        "Clean+No Dups" <- w716
        n243 = call "channelGraphs.vi"("error in (no error)"=w717, "Clean+No Dups"=w716) -> ("error out"=w722:errorcluster, "Noisy Pixel List"=→"Noisy Pixel List":i32[][], "Intensity Graph"=→"Intensity Graph":u32[][], "Detector Surface"=→"Detector Surface":refnum<class "3D Plot Datatype.lvclass">[], "Event Count Histogram"=→"Event Count Histogram":T2)  [unwired: 5 in]
        n244 = call "addStatesToQueue.vi"("State(s) in Front (\"\")"="UART Comm: Close", "State(s) in (\"\")"=w734) -> ("States Out"=w733:string)  [unwired: 13 in]
      }
      frame "---------- Pixel Status ----------" {
        # "Pixel Status Separator"
        n245 = call "addStatesToQueue.vi"("State(s) in (\"\")"=w740) -> ("States Out"=w739:string)  [unwired: 14 in]
      }
      frame "Pixel Status: Pix Send On" {
        # "Sends the command to the FPGA to toggle the status of the Pixel"
        n246 = Number To Hexadecimal String(1:i16 2 ("width (-)"), 2:"Choose Pixel") -> (0:w754:string)
        n247 = Equal To 0?(x="Select CZT") -> (x = 0?=w744:bool)
        n248 = call "hexStrConv.vi"("Input ASCII Hex String"=w754, "error in (no error)"=w747) -> ("Output Non Printable HEX String"=w753:string, "error out"=w749:errorcluster)  [unwired: 1 out]
        n249 = Select(t="Ð", s=w744, f="Ò") -> (s? t:f=w741:string)
        n250 = Concatenate Strings(w741, w753, "U") -> (w750:string)
        n251 = VISA Write(VISA resource name=w756, write buffer=w750, error in (no error)=w749) -> (VISA resource name out=w751:refnum<visa-resource-name>, error out=w748:errorcluster)  [unwired: 1 out]
        n252 = call "addStatesToQueue.vi"("State(s) in (\"\")"=w760) -> ("States Out"=w759:string)  [unwired: 14 in]
      }
      frame "Pixel Status: Pix Send Off" {
        # "Sends the command to the FPGA to toggle the status of the Pixel"
        n253 = property on="Choose Pixel" class="DigNum (strict)"(error in=w772) -> (error out=w770:errorcluster, "Value"=w771:u8)  [unwired: 1 in, 1 out]
        n254 = Number To Hexadecimal String(1:i16 2 ("width (-)"), 2:w771) -> (0:w777:string)
        n255 = call "hexStrConv.vi"("Input ASCII Hex String"=w777, "error in (no error)"=w770) -> ("Output Non Printable HEX String"=w776:string, "error out"=w765:errorcluster)  [unwired: 1 out]
        n256 = property on="Select CZT" class="RadioBtnsControl (strict)"(error in=w765) -> (error out=w764:errorcluster, "Value"=w762:enum32{"CZT 1", "CZT 2"})  [unwired: 1 in, 1 out]
        n257 = Equal To 0?(x=w762) -> (x = 0?=w767:bool)
        n258 = Select(t="Ñ", s=w767, f="Ó") -> (s? t:f=w763:string)
        n259 = Concatenate Strings(w763, w776, "U") -> (w773:string)
        n260 = VISA Write(VISA resource name=w778, write buffer=w773, error in (no error)=w764) -> (VISA resource name out=w774:refnum<visa-resource-name>, error out=w768:errorcluster)  [unwired: 1 out]
        n261 = call "addStatesToQueue.vi"("State(s) in (\"\")"=w782) -> ("States Out"=w781:string)  [unwired: 14 in]
      }
      frame "Pixel Status: Pix Rec" {
        # "Recieves the data from the FPGA whether the operation has been sucessfully performed or not"
        n262 = VISA Read(VISA resource name=w802, byte count=u32 16, error in (no error)=w800) -> (VISA resource name out=w801:refnum<visa-resource-name>, read buffer=w796:string, error out=w793:errorcluster)  [unwired: 1 out]
        n263 = call <vilib>:"Trim Whitespace.vi"("string"=w796) -> ("trimmed string"=w791:string)  [unwired: 1 in]
        n264 = call "pixStatusConvert.vi"("format string"="D%1x%2x", "error in"=w793, "Hex Input String"=w791) -> ("error out"=w790:errorcluster, "Pix No."=w792:u16, "En/Dis?"=w794:bool)  [unwired: 6 in]
        n265 = property on="Select CZT" class="RadioBtnsControl (strict)"(error in=w790) -> (error out=w789:errorcluster, "Value"=w787:enum32{"CZT 1", "CZT 2"})  [unwired: 1 in, 1 out]
        n266 = Equal To 0?(x=w787) -> (x = 0?=w786:bool)
        n267 = case shown="False" w786 {
          tunnel: [w809 w813] -> w799
          tunnel: w798 -> [w808 w812]
          tunnel: w794 -> [w807 w811]
          tunnel: w792 -> [w806 w810]
          frame False {
            n268 = Bundle By Name(cluster=w808, "Pixel Status 2.Pixel En/Dis?"=w807, "Pixel Status 2.Pixel Number"=w806) -> (w809:T9)
          }
          frame True {
            n269 = Bundle By Name(cluster=w812, "Pixel Status 1.Pixel En/Dis?"=w811, "Pixel Status 1.Pixel Number"=w810) -> (w813:T9)
          }
        }
        n270 = Select(t=enum32{"CZT 1", "CZT 2"}."CZT 1" ("Tab Control 2"), s=w786, f=enum32{"CZT 1", "CZT 2"}."CZT 2" ("Tab Control 2")) -> (s? t:f=w783:enum32{"CZT 1", "CZT 2"})
        n271 = property on="CZT Tabs" class="TabCtl (strict)"(error in=w789, "Value"=w783) -> (error out=w788:errorcluster)  [unwired: 1 in, 1 out]
        n272 = call "addStatesToQueue.vi"("State(s) in (\"\")"=w805) -> ("States Out"=w804:string)  [unwired: 14 in]
      }
      frame "Pixel Status: Update Pix Matrix" {
        # "Updates the Pixel matrix UI"
        n273 = property on="Select CZT" class="RadioBtnsControl (strict)"(error in=w818) -> (error out=w817:errorcluster, "Value"=w814:enum32{"CZT 1", "CZT 2"})  [unwired: 1 in, 1 out]
        n274 = case shown="\"CZT 1\"" w814 {
          tunnel: w820 -> [w825 w836 w847]
          tunnel: [w826 w838 w847] -> w819
          tunnel: w816 -> [w834 w835 w846]
          tunnel: [w834 w835 w846] -> w815
          frame "CZT 1" {
            n275 = Unbundle By Name(w825) -> ("Pixel Status 1.Pixel Array"=w833:bool[][], "Pixel Status 1.Pixel Number"=w829:u16, "Pixel Status 1.Pixel En/Dis?"=w830:bool, "Pixel Status 1"=w828:T10)
            n276 = call "noToCoord.vi"("Pixel number"=w829) -> ("i"=w832:u8, "j"=w831:u8)  [unwired: 6 in]
            n277 = Replace Array Subset(array=w833, new element=w830, index (row)=w832, index (col)=w831) -> (w824:bool[][])
            "Pixel Status 1" <- w824
            n278 = call "addRemDisList.vi"("Pixel Status"=w828) -> ("Disabled Pixels"=w827:u8[])  [unwired: 10 in]
            n279 = Bundle By Name(cluster=w825, "Pixel Status 1.Pixel Array"=w824, "Pixel Status 1.Disabled Pixels"=w827) -> (w826:T9)
          }
          frame "CZT 2" {
            n280 = Unbundle By Name(w836) -> ("Pixel Status 2.Pixel Array"=w845:bool[][], "Pixel Status 2.Pixel Number"=w840:u16, "Pixel Status 2.Pixel En/Dis?"=w841:bool, "Pixel Status 2"=w839:T10)
            n281 = call "noToCoord.vi"("Pixel number"=w840) -> ("i"=w844:u8, "j"=w843:u8)  [unwired: 6 in]
            n282 = Replace Array Subset(array=w845, new element=w841, index (row)=w844, index (col)=w843) -> (w842:bool[][])
            "Pixel Status 2" <- w842
            n283 = call "addRemDisList.vi"("Pixel Status"=w839) -> ("Disabled Pixels"=w837:u8[])  [unwired: 10 in]
            n284 = Bundle By Name(cluster=w836, "Pixel Status 2.Pixel Array"=w842, "Pixel Status 2.Disabled Pixels"=w837) -> (w838:T9)
          }
          frame Default {
          }
        }
        n285 = call "addStatesToQueue.vi"("State(s) in (\"\")"=w823) -> ("States Out"=w822:string)  [unwired: 14 in]
      }
      frame "---------- All Pixel Status ----------" {
        # "All Pixel Status Separator"
        n286 = call "addStatesToQueue.vi"("State(s) in (\"\")"=w853) -> ("States Out"=w852:string)  [unwired: 14 in]
      }
      frame "All Pixel Status: Pix Send All" {
        n287 = VISA Write(VISA resource name=w858, write buffer="ß\u0000U", error in (no error)=w856) -> (VISA resource name out=w857:refnum<visa-resource-name>, error out=w855:errorcluster)  [unwired: 1 out]
        n288 = call "addStatesToQueue.vi"("State(s) in (\"\")"=w862) -> ("States Out"=w861:string)  [unwired: 14 in]
      }
      frame "All Pixel Status: Pix Rec All" {
        w868 = "D%1x%2x" ("format string")
        n289 = VISA Read(VISA resource name=w881, byte count=u32 32, error in (no error)=w880) -> (VISA resource name out=w882:refnum<visa-resource-name>, read buffer=w869:string, error out=w872:errorcluster)  [unwired: 1 out]
        n290 = call <vilib>:"Trim Whitespace.vi"("string"=w869) -> ("trimmed string"=w865:string)  [unwired: 1 in]
        n291 = call "dataSplitter.vi"("Input"=w865) -> ("After \\t"=w863:string, "Before \\t"=w864:string)  [unwired: 2 in]
        n292 = call "pixStatusConvert.vi"("format string"=w868, "error in"=w872, "Hex Input String"=w864) -> ("error out"=w873:errorcluster, "Pix No."=w875:u16, "En/Dis?"=w876:bool)  [unwired: 6 in]
        n293 = call "pixStatusConvert.vi"("format string"=w868, "error in"=w872, "Hex Input String"=w863) -> ("error out"=w874:errorcluster, "Pix No."=w866:u16, "En/Dis?"=w867:bool)  [unwired: 6 in]
        n294 = Bundle By Name(cluster=w879, "Pixel Status 1.Pixel En/Dis?"=w876, "Pixel Status 1.Pixel Number"=w875, "Pixel Status 2.Pixel En/Dis?"=w867, "Pixel Status 2.Pixel Number"=w866) -> (w878:T9)
        n295 = Merge Errors(w873, w874) -> (w871:errorcluster)
        n296 = call "addStatesToQueue.vi"("State(s) in Front (\"\")"="All Pixel Status: Update Matrix", "State(s) in (\"\")"=w885) -> ("States Out"=w884:string)  [unwired: 13 in]
      }
      frame "All Pixel Status: Update Matrix" {
        n297 = Unbundle By Name(w905) -> ("Pixel Status 1.Pixel Array"=w906:bool[][], "Pixel Status 1.Pixel Number"=w897:u16, "Pixel Status 1.Pixel En/Dis?"=w908:bool, "Pixel Status 1"=w909:T10, "Pixel Status 2.Pixel Array"=w893:bool[][], "Pixel Status 2.Pixel Number"=w894:u16, "Pixel Status 2.Pixel En/Dis?"=w892:bool, "Pixel Status 2"=w891:T10)
        n298 = call "noToCoord.vi"("Pixel number"=w894) -> ("i"=w896:u8, "j"=w895:u8)  [unwired: 6 in]
        n299 = call "noToCoord.vi"("Pixel number"=w897) -> ("i"=w907:u8, "j"=w911:u8)  [unwired: 6 in]
        n300 = call "addRemDisList.vi"("Pixel Status"=w891) -> ("Disabled Pixels"=w890:u8[])  [unwired: 10 in]
        n301 = Replace Array Subset(array=w906, new element=w908, index (row)=w907, index (col)=w911) -> (w902:bool[][])
        n302 = call "addRemDisList.vi"("Pixel Status"=w909) -> ("Disabled Pixels"=w910:u8[])  [unwired: 10 in]
        n303 = Replace Array Subset(array=w893, new element=w892, index (row)=w896, index (col)=w895) -> (w886:bool[][])
        n304 = Bundle By Name(cluster=w905, "Pixel Status 1.Pixel Array"=w902, "Pixel Status 1.Disabled Pixels"=w910, "Pixel Status 2.Pixel Array"=w886, "Pixel Status 2.Disabled Pixels"=w890) -> (w904:T9)
        n305 = property on="Pixel Status 1" class="Arr (strict)"(error in=w903, "Value"=w902) -> (error out=w888:errorcluster)  [unwired: 1 in, 1 out]
        n306 = property on="Pixel Status 2" class="Arr (strict)"(error in=w888, "Value"=w886) -> (error out=w887:errorcluster)  [unwired: 1 in, 1 out]
        n307 = Equal?(x=w897, y=255) -> (x = y?=w901:bool)
        n308 = Select(t="UART Comm: Close", s=w901, f="All Pixel Status: Pix Rec All") -> (s? t:f=w900:string)
        n309 = call "addStatesToQueue.vi"("State(s) in Front (\"\")"=w900, "State(s) in (\"\")"=w915) -> ("States Out"=w914:string)  [unwired: 13 in]
      }
      frame "---------- Threshold ----------" {
        # "Threshold States Separator"
        n310 = call "addStatesToQueue.vi"("State(s) in (\"\")"=w921) -> ("States Out"=w920:string)  [unwired: 14 in]
      }
      frame "Threshold: Set Thresh" {
        # "Sends command to set the user selected threshold value"
        n311 = call "threshConvert.vi"("error in"=w923, "Select Threshold Value"="Select Threshold Value") -> ("error out"=w928:errorcluster, "Threshold Frame"=w926:string)  [unwired: 8 in]
        n312 = Concatenate Strings(w926, "U" ("string")) -> (w924:string)
        n313 = VISA Write(VISA resource name=w922, write buffer=w924, error in (no error)=w928) -> (VISA resource name out=w929:refnum<visa-resource-name>, error out=w927:errorcluster)  [unwired: 1 out]
        n314 = call "addStatesToQueue.vi"("State(s) in (\"\")"=w934) -> ("States Out"=w933:string)  [unwired: 14 in]
      }
      frame "Threshold: Get Thresh" {
        w940 = "E%x" ("format string")
        # "Reads the value of the updated threshold energy"
        n315 = VISA Read(VISA resource name=w951, byte count=u32 16, error in (no error)=w949) -> (VISA resource name out=w950:refnum<visa-resource-name>, read buffer=w937:string, error out=w944:errorcluster)  [unwired: 1 out]
        n316 = call "dataSplitter.vi"("Input"=w937) -> ("After \\t"=w935:string, "Before \\t"=w936:string)  [unwired: 2 in]
        n317 = call "getThreshConv.vi"("format string"=w940, "error in (no error)"=w944, "Input HEX Threshold"=w935) -> ("error out"=w942:errorcluster, "Output Threshold Value"=→"CZT 2 Thresh":u16)  [unwired: 6 in, 1 out]
        n318 = call "getThreshConv.vi"("format string"=w940, "error in (no error)"=w944, "Input HEX Threshold"=w936) -> ("error out"=w943:errorcluster, "Output Threshold Value"=→"CZT 1 Thresh":u16)  [unwired: 6 in, 1 out]
        n319 = Merge Errors(w943, w942) -> (w941:errorcluster)
        n320 = Select(t="", s=w941, f=w945) -> (s? t:f=w946:string)
        n321 = call "addStatesToQueue.vi"("State(s) in Front (\"\")"=w946, "State(s) in (\"\")"=w955) -> ("States Out"=w954:string)  [unwired: 13 in]
      }
      frame "---------- Serial Number ----------" {
        # "Serial Number States Separator"
        n322 = call "addStatesToQueue.vi"("State(s) in (\"\")"=w961) -> ("States Out"=w960:string)  [unwired: 14 in]
      }
      frame "Serial Number: Send Command" {
        # "Send command to read serial number from CZT"
        n323 = call "hexStrConv.vi"("Input ASCII Hex String"="B000" ("format string"), "error in (no error)"=w964) -> ("Output Non Printable HEX String"=w962:string, "error out"=w963:errorcluster)  [unwired: 1 out]
        n324 = Concatenate Strings(w962, "U" ("string")) -> (w967:string)
        n325 = VISA Write(VISA resource name=w966, write buffer=w967, error in (no error)=w963) -> (VISA resource name out=w970:refnum<visa-resource-name>, error out=w969:errorcluster)  [unwired: 1 out]
        n326 = call "addStatesToQueue.vi"("State(s) in (\"\")"=w974) -> ("States Out"=w973:string)  [unwired: 14 in]
      }
      frame "Serial Number: Get Number" {
        w979 = u32 0 ("default (0 U32)")
        # "Template Separator\n(You can make a copy of, or modify, this frame)"
        # "Recieve the v"
        n327 = VISA Read(VISA resource name=w992, byte count=u32 16, error in (no error)=w990) -> (VISA resource name out=w991:refnum<visa-resource-name>, read buffer=w978:string, error out=w989:errorcluster)  [unwired: 1 out]
        n328 = call "dataSplitter.vi"("Input"=w978) -> ("After \\t"=w976:string, "Before \\t"=w977:string)  [unwired: 2 in]
        n329 = String Subset(string=w976, offset (0)=1) -> (substring=w982:string)  [unwired: 1 in]
        n330 = String Subset(string=w977, offset (0)=1) -> (substring=w984:string)  [unwired: 1 in]
        n331 = Hexadecimal String To Number(string=w982, default (0uL)=w979) -> (number=→"CZT 2 Serial":u32)  [unwired: 1 in, 1 out]
        n332 = Hexadecimal String To Number(string=w984, default (0uL)=w979) -> (number=→"CZT 1 Serial":u32)  [unwired: 1 in, 1 out]
        n333 = Select(t="", s=w989, f=w986) -> (s? t:f=w987:string)
        n334 = call "addStatesToQueue.vi"("State(s) in Front (\"\")"=w987, "State(s) in (\"\")"=w996) -> ("States Out"=w995:string)  [unwired: 13 in]
      }
      frame "Serial Number: Verify Number" {
        n335 = property on="CZT 1 Serial" class="DigNum (strict)"(error in=w1005) -> (error out=w1001:errorcluster, "Value"=w1003:sgl)  [unwired: 1 in, 1 out]
        n336 = Equal?(x="CZT 1 Serial In", y=w1003) -> (x = y?=→"Serial1 Same?":bool)
        n337 = property on="CZT 2 Serial" class="DigNum (strict)"(error in=w1001) -> (error out=w997:errorcluster, "Value"=w999:sgl)  [unwired: 1 in, 1 out]
        n338 = Equal?(x="CZT 2 Serial In", y=w999) -> (x = y?=→"Serial2 Same?":bool)
        n339 = Select(t="", s=w997, f=w1007) -> (s? t:f=w1008:string)
        n340 = call "addStatesToQueue.vi"("State(s) in Front (\"\")"=w1008, "State(s) in (\"\")"=w1013) -> ("States Out"=w1012:string)  [unwired: 13 in]
      }
      frame "---------- Clock ----------" {
        # "Clock Freq States Separator"
        n341 = call "addStatesToQueue.vi"("State(s) in (\"\")"=w1019) -> ("States Out"=w1018:string)  [unwired: 14 in]
      }
      frame "Clock: Set Clock" {
        n342 = Number To Hexadecimal String(1:i16 2 ("width (-)"), 2:"Set CZT Clock") -> (0:w1021:string)
        n343 = call "hexStrConv.vi"("Input ASCII Hex String"=w1021, "error in (no error)"=w1026) -> ("Output Non Printable HEX String"=w1024:string, "error out"=w1025:errorcluster)  [unwired: 1 out]
        n344 = Concatenate Strings("À", w1024, "U" ("string")) -> (w1028:string)
        n345 = VISA Write(VISA resource name=w1027, write buffer=w1028, error in (no error)=w1025) -> (VISA resource name out=w1031:refnum<visa-resource-name>, error out=w1030:errorcluster)  [unwired: 1 out]
        n346 = call "addStatesToQueue.vi"("State(s) in (\"\")"=w1035) -> ("States Out"=w1034:string)  [unwired: 14 in]
      }
      frame "Clock: Get Clock" {
        n347 = VISA Read(VISA resource name=w1057, byte count=u32 16, error in (no error)=w1055) -> (VISA resource name out=w1056:refnum<visa-resource-name>, read buffer=w1038:string, error out=w1054:errorcluster)  [unwired: 1 out]
        n348 = call "dataSplitter.vi"("Input"=w1038) -> ("After \\t"=w1036:string, "Before \\t"=w1037:string)  [unwired: 2 in]
        n349 = String Subset(string=w1036, offset (0)=1) -> (substring=w1047:string)  [unwired: 1 in]
        n350 = String Subset(string=w1037, offset (0)=1) -> (substring=w1050:string)  [unwired: 1 in]
        n351 = Hexadecimal String To Number(string=w1047, default (0uL)=u32 0 ("default (0 U32)")) -> (number=w1040:u32)  [unwired: 1 in, 1 out]
        n352 = Hexadecimal String To Number(string=w1050) -> (number=w1044:u32)  [unwired: 2 in, 1 out]
        n353 = Multiply(x=w1044, y=u8 5) -> (x*y=→"CZT 1\nFrequency":u32)
        n354 = Multiply(x=w1040, y=u8 5) -> (x*y=→"CZT 2 \nFrequency":u32)
        n355 = Select(t="", s=w1054, f=w1051) -> (s? t:f=w1052:string)
        n356 = call "addStatesToQueue.vi"("State(s) in Front (\"\")"=w1052, "State(s) in (\"\")"=w1061) -> ("States Out"=w1060:string)  [unwired: 13 in]
      }
      frame "---------- EEPROM ----------" {
        # "EEPROM States Separator"
        n357 = call "addStatesToQueue.vi"("State(s) in (\"\")"=w1067) -> ("States Out"=w1066:string)  [unwired: 14 in]
      }
      frame "EEPROM: Update" {
        n358 = VISA Write(VISA resource name=w1070, write buffer="ð\u0001U", error in (no error)=w1068) -> (VISA resource name out=w1072:refnum<visa-resource-name>, error out=w1071:errorcluster)  [unwired: 1 out]
        n359 = call "addStatesToQueue.vi"("State(s) in (\"\")"=w1076) -> ("States Out"=w1075:string)  [unwired: 14 in]
      }
      frame "EEPROM: Reset" {
        n360 = VISA Write(VISA resource name=w1079, write buffer="ð\u0000U", error in (no error)=w1078) -> (VISA resource name out=w1081:refnum<visa-resource-name>, error out=w1080:errorcluster)  [unwired: 1 out]
        n361 = call "addStatesToQueue.vi"("State(s) in (\"\")"=w1085) -> ("States Out"=w1084:string)  [unwired: 14 in]
      }
      frame "---------- UART Comm ----------" {
        # "UART Communication Separator"
        n362 = call "addStatesToQueue.vi"("State(s) in (\"\")"=w1091) -> ("States Out"=w1090:string)  [unwired: 14 in]
      }
      frame "UART Comm: Init" {
        # "Initialize the UART communication settings"
        n363 = disable-structure shown="Enabled" {
          disable-tunnel: [w1112 T1 {"VISA resource name"="COM6", "baud rate"=115200, "data bits"=8, "parity"=enum."None", "stop bits"=10, "flow control"=0} ("Serial Settings") "Serial Settings"] -> w1107
          frame Disabled {
            n364 = global read "serialSettings_Global.vi" "Serial Settings"() -> (w1112:T1)
          }
          frame Disabled {
          }
          frame Enabled {
          }
        }
        n365 = Unbundle(w1107) -> ("VISA resource name"=w1106:refnum<visa-resource-name>, "baud rate"=w1105:u32, "data bits"=w1104:u16, "parity"=w1103:enum16{"None", "Odd", "Even", "Mark", "Space"}, "stop bits"=w1102:u16, "flow control"=w1101:u16)
        n366 = call-poly "VISA Configure Serial Port"("VISA resource name"=w1106, "timeout (10sec)"=u32 1000, "termination char\n(0xA = '\\n' = LF)"=u8 10 ("termination char\n(0xA = '\\n' = LF)"), "Enable Termination\nChar (T)"=TRUE ("Enable Termination\nChar (T)"), "baud rate (9600)"=w1105, "data bits (8)"=w1104, "parity (0:none)"=w1103, "error in (no error)"=w1108, "stop bits (10: 1 bit)"=w1102, "flow control (0:none)"=w1101) -> ("VISA resource name out"=w1096:refnum<visa-resource-name>, "error out"=w1095:errorcluster)  [unwired: 4 in]
        n367 = Select(t="", s=w1095, f=w1097) -> (s? t:f=w1100:string)
        n368 = call "addStatesToQueue.vi"("State(s) in Front (\"\")"=w1100, "State(s) in (\"\")"=w1111) -> ("States Out"=w1110:string)  [unwired: 13 in]
      }
      frame "UART Comm: Close" {
        w1121 = T16 128 items=["Flush Receive Buffer"=16, "Write Transmit Buffer to Device"=32, "Flush Receive Buffer (No I/O)"=64, "Flush Transmit Buffer"=128] ("Mask")
        w1120 = T16 16 items=["Flush Receive Buffer"=16, "Write Transmit Buffer to Device"=32, "Flush Receive Buffer (No I/O)"=64, "Flush Transmit Buffer"=128] ("Mask")
        # "Closes the reference to UART"
        n369 = Or(x=w1120, y=w1121) -> (x .or. y?=w1119:T16)
        n370 = VISA Flush I/O Buffer(VISA resource name=w1125, mask (16)=w1119, error in (no error)=w1123) -> (VISA resource name out=w1124:refnum<visa-resource-name>, error out=w1122:errorcluster)
        n371 = VISA Close(VISA resource name=w1124, error in (no error)=w1122) -> (error out=w1117:errorcluster)
        n372 = Select(t="", s=w1117, f=w1116) -> (s? t:f=w1115:string)
        n373 = call "addStatesToQueue.vi"("State(s) in Front (\"\")"=w1115, "State(s) in (\"\")"=w1129) -> ("States Out"=w1128:string)  [unwired: 13 in]
      }
    }
    "States Left" <- w18
  }
  "Exit error code" <- w5
  n374 = while {
    tunnel: w4 -> [w1131]
    stop <- w1130 stop-if-true
    # "Clock Display Loop"
    n375 = Get Date/Time In Seconds() -> (seconds since 1Jan1904=→"Current Time":timestamp)
    n376 = call <extravilib>:"Read.vi"("channel"=w1131) -> ("element"=w1130:bool)  [unwired: 1 in, 1 out]
    n377 = Wait (ms)(milliseconds to wait=u32 100) -> ()  [unwired: 1 out]
  }
